vi "AbelFcsMain.vi"() -> ()   [LabVIEW 2009]
uses:
  Camera/vi/ccdChipPixels.vi
  Camera/vi/GlobalSetGetConfigureCamera.vi
  Camera/lib/System Files/user.lib/atmcd32d.llb/Shutter_mode typedef.ctl
  Camera/lib/System Files/user.lib/atmcd32d.llb/Shutter_type typedef.ctl
  Variables/GetPicture.vi
  Camera/vi/StopGetPic.vi
  Camera/vi/CamDef.vi
  Variables/GlobalLaserInterface.vi
  Variables/patternImg.vi
  <vilib>/vision/Image Controls.llb/IMAQ Rounding Mode.ctl
  Variables/GlobalConAxisPI.vi
  Variables/GlobalCameraHandle.vi
  <vilib>/vision/Pattern Matching.llb/IMAQ Match Range Setting.ctl
  <vilib>/vision/Pattern Matching.llb/IMAQ Curve Parameters.ctl
panel:
  out "subarray":dbl[](array[numeric])
  in  "Settings (GeometricMatching)":T3 {"Curve Parameters"."Extraction Mode" items=["Normal", "Uniform Regions"]; "Curve Parameters"."Edge Filter Size" items=["Fine", "Normal", "Contour Tracing"]; "Curve Parameters"."Max Endpoint Gap" min=0; "Curve Parameters"."Col Search Step Size" min=1 max=255 step=1; "Curve Parameters"."Row Search Step Size" min=1 max=255 step=1; "Curve Parameters"."Min Length" min=0; "Curve Parameters"."Edge Threshold" min=1 max=350 step=1; "Range Settings"."Max" format="%.2f"; "Range Settings"."Min" format="%.2f"; "Range Settings"."Match Constraints" items=["Rotation Angle (degrees)", "Scale Factor (%)", "Occlusion (%)"]; "Adv. Geometric Match Options 2"."Setup Data Item" items=["Curve Extraction Mode", "Curve Edge Threshold", "Curve Edge Filter Size", "Min Curve Length", "Curve Row Search Step Size", "Curve Col Search Step Size", "Curve Max Endpoint Gap", "Extract Closed Curves", "Enable Subpixel Curve Extraction", "Enable Correlation Score", "Enable Subpixel Accuracy", "Subpixel Iterations", "Subpixel Tolerance", "Initial Match List Length", "Enable Target Template Curve Score", "Min Match Separation Distance", "Min Match Separation Angle", "Min Match Separation Scale", "Max Match Overlap", "Enable Coarse Result", "Enable Calibration Support", "Enable Contrast Reversal", "Search Strategy", "Refinement Match Factor", "Subpixel Match Factor"]}
  in  "Tab Control":T4(tab)
  out "Histogram":i32[][](graph)
  out "Trace":i32[][](graph)
  out "Point":dbl[][](graph)
  out "Image Out":T5(plugin-control)
  out "Image Number":u32
  out "acquired FPS":dbl
  out "Image":i32[][](graph)
  out "AM image":T5(plugin-control)
  out "Number of Particles":i32
  out "Image 2":dbl[][](graph)
  out "Auto Measure Points":i32
  out "NxtAutMesPoint":i32
  out "Pattern":dbl[][](array[numeric])
  out "X Steps":dbl
  out "3dAbelFcs":bool
  out "Y Steps":dbl
  out "Z Steps":dbl
  out "concatenated string":string
  out "Global Stop":bool
  out "Stop Measurement":bool
  in  "DeviceTabs":T6(tab)
  in  "WS File Tree":string(tree)
  out "Workspace":path
  in  "New MSW":bool
  in  "Open MSW":bool
  in  "Sample description":string
  in  "Save Files":bool
  out "Last Image File No":i32
  in  "Get Position":bool
  in  "Move Stage":bool
  in  "X-Position":dbl caption="X" min=0.0 max=200.0 step=0.1 format="%1.3f um"
  in  "Y-Position":dbl caption="Y" min=0.0 max=200.0 step=0.1 format="%1.3f um"
  in  "Z-Position":dbl caption="Z" min=0.0 max=200.0 step=0.1 format="%1.3f um"
  out "x-position":dbl format="%.3f"
  out "y-position":dbl format="%.3f"
  out "z-position":dbl format="%.3f"
  in  "CFD Settings":T7
  in  "Laser  Profile":string
  in  "Auto Exposure::Mode":u32(ring) items=["Relative", "Ignored"]
  in  "Brightness::Mode":u32(ring) items=["Relative", "Ignored"]
  in  "Gain::Mode":u32(ring) items=["Absolute", "Auto", "Relative", "Ignored"]
  in  "Gamma::Mode":u32(ring) items=["Relative", "Off", "Ignored"]
  in  "Shutter::Mode":u32(ring) items=["Auto", "Relative", "Ignored"]
  in  "Trigger::Trigger Activation":u32(ring) items=["Level Low", "Level High"]
  in  "Trigger::Trigger Mode":u32(ring) items=["Mode 0", "Mode 1", "Mode 15", "Off"]
  in  "Trigger Delay::Mode":u32(ring) items=["Absolute", "Relative", "Off", "Ignored"]
  in  "Brightness::Value":dbl min=0.0 max=1023.0 step=1.0
  in  "Shutter::Value":dbl min=1.0 max=4095.0 step=1.0
  in  "Auto Exposure::Value":dbl min=50.0 max=205.0 step=1.0
  in  "Gain::Value":dbl min=0.0 max=680.0 step=1.0
  in  "Trigger::Trigger Parameter":u32 max=0
  in  "Get Temperature":bool
  in  "SET CCD":bool
  in  "OPEN SHUTER":bool
  in  "Close":bool
  in  "Gain":bool
  in  "Start":bool
  in  "Stop":bool
  in  "Exposure":bool
  in  "Set Temperature":bool
  in  "duty cycle":dbl format="%.6f"
  in  "frequency":dbl format="%.6f"
  in  "PI SystemNumber":i32
  in  "Image Measurent Parameters":T8
  in  "Measurement Tab Control":T9(tab)
  in  "SCANNER EMERGENCY":bool
  in  "Stop Program":bool
  out "Task":T10(ring)
  in  "Point Defocussed Cam":bool
  in  "Adjustment":bool
  in  "Laser pulse duration":i32[](array[numeric]) min=2 max=100000 step=1 format="%d µs"
  in  "Measurement Time":i32 min=10 format="%.0d s"
  in  "Point Measurement":bool
  out "Counts":u32[](array[numeric])
  in  "Axis":enum32{"x-y", "x-z", "y-x", "y-z", "z-x", "z-y"}(ring)
  in  "Picture size 2":dbl min=0.1 max=200.0 format="%1.1f um"
  in  "Picture size":dbl min=0.1 max=200.0 format="%1.1f um"
  in  "Pixel time":dbl min=0.1 max=100.0 step=0.1 format="%.1f ms"
  in  "Resolution":dbl min=0.01 max=10.0 step=0.01 format="%.2f µm"
  out "Measure. time":dbl format="%7.1f s"
  in  "Aquire Image":bool
  out "y":i16
  out "x":i16
  in  "Save Color Image":bool
  in  "Cam (Defocused)":bool
  in  "How long?":bool
  out "Estimated Time (h)":dbl
  in  "Mesaurement Time (Sec) / Step":dbl
  in  "Start 3D FCS Abel Scan":bool
  in  "FCS Point Measurement":bool
  in  "Z Stepsize":dbl
  in  "Y Stepsize":dbl
  in  "X Stepsize":dbl
  in  "Z End":dbl
  in  "Y End":dbl
  in  "X End":dbl
  in  "Z Start":dbl
  in  "Y Start":dbl
  in  "X Start":dbl
  in  "Find Mols":bool
  in  "Filter":bool
  in  "Remove Outliers":i32
  in  "Exclude / Include X":bool
  in  "X Start 2":dbl
  in  "X End 2":dbl
  in  "Exclude / Include Y":bool
  in  "Y Start 2":dbl
  in  "Y End 2":dbl
  in  "Measurement Parameter 1":T11 items=["Center of Mass X", "Center of Mass Y", "First Pixel X", "First Pixel Y", "Bounding Rect Left", "Bounding Rect Top", "Bounding Rect Right", "Bounding Rect Bottom", "Max Feret Diameter Start X", "Max Feret Diameter Start Y", "Max Feret Diameter End X", "Max Feret Diameter End Y", "Max Horiz. Segment Length Left", "Max Horiz. Segment Length Right", "Max Horiz. Segment Length Row", "-", "Bounding Rect Width", "Bounding Rect Height", "Bounding Rect Diagonal", "Perimeter", "Convex Hull Perimeter", "Holes' Perimeter", "Max Feret Diameter", "Equivalent Ellipse Major Axis", "Equivalent Ellipse Minor Axis", "Equivalent Ellipse Minor Axis (Feret)", "Equivalent Rect Long Side", "Equivalent Rect Short Side", "Equivalent Rect Diagonal", "Equivalent Rect Short Side (Feret)", "Average Horiz. Segment Length", "Average Vert. Segment Length", "Hydraulic Radius", "Waddel Disk Diameter", "-", "Area", "Holes' Area", "Particle & Holes' Area", "Convex Hull Area", "Image Area", "-", "Number of Holes", "Number of Horiz. Segments", "Number of Vert. Segments", "-", "Orientation", "Max Feret Diameter Orientation", "-", "% Area/Image Area", "% Area/(Particle & Holes' Area)", "Ratio of Equivalent Ellipse Axes", "Ratio of Equivalent Rect Sides", "-", "Elongation Factor", "Compactness Factor", "Heywood Circularity Factor", "Type Factor", "-", "Sum X", "Sum Y", "Sum XX", "Sum XY", "Sum YY", "Sum XXX", "Sum XXY", "Sum XYY", "Sum YYY", "-", "Moment of Inertia XX", "Moment of Inertia XY", "Moment of Inertia YY", "Moment of Inertia XXX", "Moment of Inertia XXY", "Moment of Inertia XYY", "Moment of Inertia YYY", "Norm. Moment of Inertia XX", "Norm. Moment of Inertia XY", "Norm. Moment of Inertia YY", "Norm. Moment of Inertia XXX", "Norm. Moment of Inertia XXY", "Norm. Moment of Inertia XYY", "Norm. Moment of Inertia YYY", "Hu Moment 1", "Hu Moment 2", "Hu Moment 3", "Hu Moment 4", "Hu Moment 5", "Hu Moment 6", "Hu Moment 7"]
  in  "Range Lower Value Par 1":dbl
  in  "Range Upper Value  Par 1":dbl
  in  "Ex/In Par 1":bool
  in  "Measurement Parameter 2":T11 items=["Center of Mass X", "Center of Mass Y", "First Pixel X", "First Pixel Y", "Bounding Rect Left", "Bounding Rect Top", "Bounding Rect Right", "Bounding Rect Bottom", "Max Feret Diameter Start X", "Max Feret Diameter Start Y", "Max Feret Diameter End X", "Max Feret Diameter End Y", "Max Horiz. Segment Length Left", "Max Horiz. Segment Length Right", "Max Horiz. Segment Length Row", "-", "Bounding Rect Width", "Bounding Rect Height", "Bounding Rect Diagonal", "Perimeter", "Convex Hull Perimeter", "Holes' Perimeter", "Max Feret Diameter", "Equivalent Ellipse Major Axis", "Equivalent Ellipse Minor Axis", "Equivalent Ellipse Minor Axis (Feret)", "Equivalent Rect Long Side", "Equivalent Rect Short Side", "Equivalent Rect Diagonal", "Equivalent Rect Short Side (Feret)", "Average Horiz. Segment Length", "Average Vert. Segment Length", "Hydraulic Radius", "Waddel Disk Diameter", "-", "Area", "Holes' Area", "Particle & Holes' Area", "Convex Hull Area", "Image Area", "-", "Number of Holes", "Number of Horiz. Segments", "Number of Vert. Segments", "-", "Orientation", "Max Feret Diameter Orientation", "-", "% Area/Image Area", "% Area/(Particle & Holes' Area)", "Ratio of Equivalent Ellipse Axes", "Ratio of Equivalent Rect Sides", "-", "Elongation Factor", "Compactness Factor", "Heywood Circularity Factor", "Type Factor", "-", "Sum X", "Sum Y", "Sum XX", "Sum XY", "Sum YY", "Sum XXX", "Sum XXY", "Sum XYY", "Sum YYY", "-", "Moment of Inertia XX", "Moment of Inertia XY", "Moment of Inertia YY", "Moment of Inertia XXX", "Moment of Inertia XXY", "Moment of Inertia XYY", "Moment of Inertia YYY", "Norm. Moment of Inertia XX", "Norm. Moment of Inertia XY", "Norm. Moment of Inertia YY", "Norm. Moment of Inertia XXX", "Norm. Moment of Inertia XXY", "Norm. Moment of Inertia XYY", "Norm. Moment of Inertia YYY", "Hu Moment 1", "Hu Moment 2", "Hu Moment 3", "Hu Moment 4", "Hu Moment 5", "Hu Moment 6", "Hu Moment 7"]
  in  "Range Lower Value Par 2":dbl
  in  "Range Upper Value Par 2":dbl
  in  "Ex/In Par 2":bool
  in  "Square/Hexa":bool
  in  "Connectivity 4/8":bool
  in  "Manual":bool
  in  "Focuswidth":dbl
  in  "Mode":enum16{"Gauss", "Radial", "Azimuthal"}(ring)
  in  "Detection Modus":u16(ring) items=["Pattern", "Heuristic"]
  in  "NA":dbl
  in  "TSH":dbl min=0.0 max=1.0 step=0.01
  in  "Auto Defocussed Cam":bool
  in  "Autopoint-Autofocus Z":bool
  in  "Auto Measurement Time (ms)":i32 caption="Measurement Time (s)" min=10
  out "Auto Meas Progress":i32(slide) caption="Point 34 / 34"
  in  "Auto Meas":bool
  out "Active pt3":path
  out "Buffer Overrun":bool
  out "Running":bool
  # "Range"
  # "Scanner Position"
  # "Point Measurement Settings"
  # "Start Experiment"
  # "Estimated Mesaurement Time"
  # "Image Scan Settings"
  # "Save as png"
  # "Pixel"
  # "Define the 3D Space and Stepwith of your Experiment"
  # "Time of the Experiment"
  # "Check What to Mesaure"
  # "Start Your Experiment here"
  # "Lifetime Mesaurement Time on each Position"
  # "Define Search Area"
  # "Define Detection Parameters"
  # "Exact Matching"
  # "Operation"
  # "Show Progress"
  # "Automated Mesaurement on Single Molecule Coordinates on the  2D Frame"
  # "Start Your Experiment here"
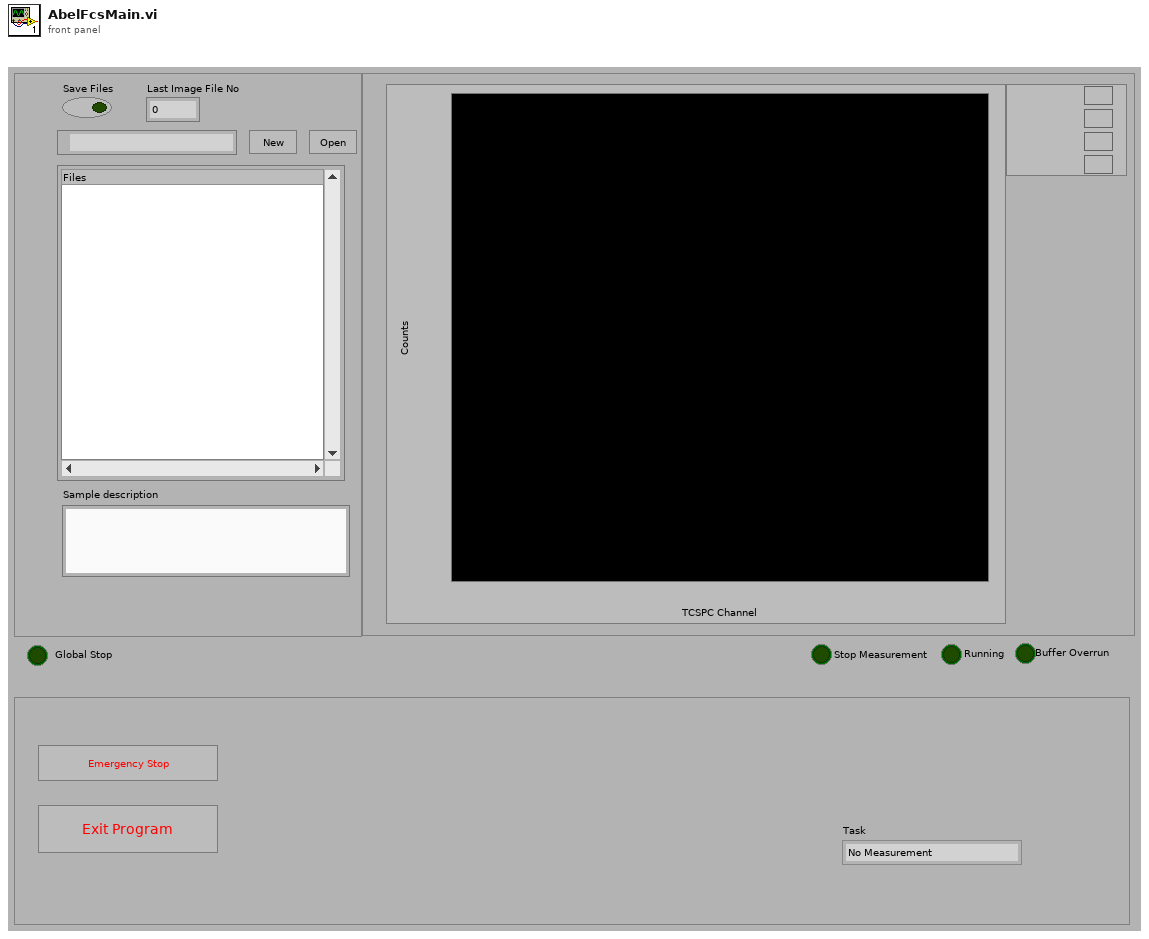
[diagram p1: front panel]
types:
  T1 = typedef "IMAQ Curve Parameters.ctl" = cluster{"Extraction Mode":u32, "Edge Threshold":i32, "Edge Filter Size":u32, "Min Length":i32, "Row Search Step Size":i32, "Col Search Step Size":i32, "Max Endpoint Gap":i32, "Closed":bool, "Subpixel":bool}
  T2 = typedef "IMAQ Match Range Setting.ctl" = cluster{"Match Constraints":u32, "Min":dbl, "Max":dbl}
  T3 = cluster{"Curve Parameters":T1, "Match Mode":cluster{"Rotation":bool, "Scale":bool, "Occlusion":bool, "Reserved":bool, "Reserved":bool, "Reserved":bool}, "Range Settings":T2[], "Number of Matches":i32, "Minimum Match Score":sgl, "SubPixel Accuracy":bool, "Adv. Geometric Match Options 2":cluster{"Setup Data Item":u16, "Item Value":dbl}[]}
  T4 = enum32{"TCSPC Histogram", "Trace", "CCD", "Backreflection", "Image", "AutoMesaurement"}
  T5 = typedef "IMAQ Image.ctl" = refnum<image>
  T6 = enum32{"Workspace", "Scanner", "HHL", "Video", "CCD", "Laser2"}
  T7 = cluster{"Sync Level":i32, "Sync ZeroX":i32, "Sync Offset":i32, "Chan Settings":cluster{"CHx Level":i32, "CHx ZeroX":i32, "CHx Offset":i32}[]}
  T8 = cluster{"Position":cluster{"X-Position":dbl, "Y-Position":dbl, "Z-Position":dbl}, "Axis 1 Pixels":dbl, "Axis 2 Pixels":dbl, "Axis":i32, "Resolution":dbl, "PixelTime":dbl, "Laser pulses":i32}
  T9 = enum32{"Main ", "Point Measurement", "Aquire Image (Area Scan)", "3D Grid FCS CCD", "Search Molecules", "AutoMode"}
  T10 = enum16{"No Measurement", "Aquire Image", "Point Measurement", "Multi Measurement", "Save Color Image", "Find Single Mol.", "Auto Measurement Control", "Auto Point", "Aquire Line Scan", "Grid Measurement", "Trapping", "Move Scanner"}
  T11 = typedef "Particle Parameters" = i32
  T12 = cluster{"Dev":i32, "SerNo":string, "HW_Model":string, "HW_Partno":string}[]
  T13 = enum16{"No Measurement", "Aquire Image", "Point Measurement", "Multi Measurement", "Save Color Image"}
  T14 = enum16{"No Measurement", "Aquire Image", "Point Measurement", "Multi Measurement", "Save Color Image", "Find Single Mol.", "Auto Measurement Control", "Auto Point"}
  T15 = enum16{"No Measurement", "Aquire Image", "Point Measurement", "Multi Measurement", "Save Color Image", "Find Single Mol."}
  T16 = enum16{"Get (Default)", "Set Workspace", "Append File", "Change Comment"}
  T17 = typedef "Shutter_type typedef.ctl" = enum16{"TTL Low", "TTL High"}
  T18 = typedef "Shutter_mode typedef.ctl" = enum16{"Auto", "Open", "Close"}
  T19 = cluster{"File No":i32, "File Path":path, "Parent File":i32, "File Type":enum16{"unknown", "pt3 File", "png Image", "bmp Image"}, "Measurement Type":enum16{"not a pt3 File", "Image File", "Point Measurement", "Auto Point", "Line Scan", "Grid Scan"}, "Upper Left":cluster{"x-Position":dbl, "y-Position":dbl, "z-Position":dbl}, "Pixels":dbl[], "Resolution":dbl, "Scan Axis":enum32{"x-y", "x-z", "y-x", "y-z", "z-x", "z-y"}, "PixelTime":dbl}[]
  T20 = cluster{"File No":i32, "File Path":path, "Parent File":i32, "File Type":enum16{"unknown", "pt3 File", "png Image", "bmp Image"}, "Measurement Type":enum16{"not a pt3 File", "Image File", "Point Measurement", "Auto Point", "Line Scan", "Grid Scan"}, "Upper Left":cluster{"x-Position":dbl, "y-Position":dbl, "z-Position":dbl}, "Pixels":i32[], "Scan Axis":enum32{"x-y", "x-z", "y-x", "y-z", "z-x", "z-y"}, "Resolution":dbl, "PixelTime":dbl}[]
  T21 = cluster{"File No":i32, "File Path":path, "Parent File":i32, "File Type":enum16{"unknown", "pt3 File", "png Image", "bmp Image"}, "Measurement Type":enum16{"not a pt3 File", "Image File", "Point Measurement", "Auto Point", "Line Scan", "Grid Scan"}, "Upper Left":cluster{"x-Position":dbl, "y-Position":dbl, "z-Position":dbl}, "Pixels":i32[], "Resolution":dbl, "Scan Axis":enum32{"x-y", "x-z", "y-z"}, "PixelTime":dbl}[]
  T22 = cluster{"Files in Workspace[0]":cluster{"File No":i32, "File Path":path, "Parent File":i32, "File Type":enum16{"unknown", "pt3 File", "png Image", "bmp Image"}, "Measurement Type":enum16{"not a pt3 File", "Image File", "Point Measurement", "Auto Point", "Line Scan", "Grid Scan"}, "Upper Left":cluster{"x-Position":dbl, "y-Position":dbl, "z-Position":dbl}, "Pixels":i32[], "Scan Axis":enum32{"x-y", "x-z", "y-x", "y-z", "z-x", "z-y"}, "Resolution":dbl, "PixelTime":dbl}, "Files in Workspace[1]":cluster{"File No":i32, "File Path":path, "Parent File":i32, "File Type":enum16{"unknown", "pt3 File", "png Image", "bmp Image"}, "Measurement Type":enum16{"not a pt3 File", "Image File", "Point Measurement", "Auto Point", "Line Scan", "Grid Scan"}, "Upper Left":cluster{"x-Position":dbl, "y-Position":dbl, "z-Position":dbl}, "Pixels":i32[], "Scan Axis":enum32{"x-y", "x-z", "y-x", "y-z", "z-x", "z-y"}, "Resolution":dbl, "PixelTime":dbl}, "Files in Workspace[2]":cluster{"File No":i32, "File Path":path, "Parent File":i32, "File Type":enum16{"unknown", "pt3 File", "png Image", "bmp Image"}, "Measurement Type":enum16{"not a pt3 File", "Image File", "Point Measurement", "Auto Point", "Line Scan", "Grid Scan"}, "Upper Left":cluster{"x-Position":dbl, "y-Position":dbl, "z-Position":dbl}, "Pixels":i32[], "Scan Axis":enum32{"x-y", "x-z", "y-x", "y-z", "z-x", "z-y"}, "Resolution":dbl, "PixelTime":dbl}, "Files in Workspace[3]":cluster{"File No":i32, "File Path":path, "Parent File":i32, "File Type":enum16{"unknown", "pt3 File", "png Image", "bmp Image"}, "Measurement Type":enum16{"not a pt3 File", "Image File", "Point Measurement", "Auto Point", "Line Scan", "Grid Scan"}, "Upper Left":cluster{"x-Position":dbl, "y-Position":dbl, "z-Position":dbl}, "Pixels":i32[], "Scan Axis":enum32{"x-y", "x-z", "y-x", "y-z", "z-x", "z-y"}, "Resolution":dbl, "PixelTime":dbl}, "Files in Workspace[4]":cluster{"File No":i32, "File Path":path, "Parent File":i32, "File Type":enum16{"unknown", "pt3 File", "png Image", "bmp Image"}, "Measurement Type":enum16{"not a pt3 File", "Image File", "Point Measurement", "Auto Point", "Line Scan", "Grid Scan"}, "Upper Left":cluster{"x-Position":dbl, "y-Position":dbl, "z-Position":dbl}, "Pixels":i32[], "Scan Axis":enum32{"x-y", "x-z", "y-x", "y-z", "z-x", "z-y"}, "Resolution":dbl, "PixelTime":dbl}, "Files in Workspace[5]":cluster{"File No":i32, "File Path":path, "Parent File":i32, "File Type":enum16{"unknown", "pt3 File", "png Image", "bmp Image"}, "Measurement Type":enum16{"not a pt3 File", "Image File", "Point Measurement", "Auto Point", "Line Scan", "Grid Scan"}, "Upper Left":cluster{"x-Position":dbl, "y-Position":dbl, "z-Position":dbl}, "Pixels":i32[], "Scan Axis":enum32{"x-y", "x-z", "y-x", "y-z", "z-x", "z-y"}, "Resolution":dbl, "PixelTime":dbl}, "Files in Workspace[6]":cluster{"File No":i32, "File Path":path, "Parent File":i32, "File Type":enum16{"unknown", "pt3 File", "png Image", "bmp Image"}, "Measurement Type":enum16{"not a pt3 File", "Image File", "Point Measurement", "Auto Point", "Line Scan", "Grid Scan"}, "Upper Left":cluster{"x-Position":dbl, "y-Position":dbl, "z-Position":dbl}, "Pixels":i32[], "Scan Axis":enum32{"x-y", "x-z", "y-x", "y-z", "z-x", "z-y"}, "Resolution":dbl, "PixelTime":dbl}, "Files in Workspace[7]":cluster{"File No":i32, "File Path":path, "Parent File":i32, "File Type":enum16{"unknown", "pt3 File", "png Image", "bmp Image"}, "Measurement Type":enum16{"not a pt3 File", "Image File", "Point Measurement", "Auto Point", "Line Scan", "Grid Scan"}, "Upper Left":cluster{"x-Position":dbl, "y-Position":dbl, "z-Position":dbl}, "Pixels":i32[], "Scan Axis":enum32{"x-y", "x-z", "y-x", "y-z", "z-x", "z-y"}, "Resolution":dbl, "PixelTime":dbl}, "Files in Workspace[8]":cluster{"File No":i32, "File Path":path, "Parent File":i32, "File Type":enum16{"unknown", "pt3 File", "png Image", "bmp Image"}, "Measurement Type":enum16{"not a pt3 File", "Image File", "Point Measurement", "Auto Point", "Line Scan", "Grid Scan"}, "Upper Left":cluster{"x-Position":dbl, "y-Position":dbl, "z-Position":dbl}, "Pixels":i32[], "Scan Axis":enum32{"x-y", "x-z", "y-x", "y-z", "z-x", "z-y"}, "Resolution":dbl, "PixelTime":dbl}}
  T23 = typedef "LVPoint32TypeDef.ctl" = cluster{"Horizontal":i32, "Vertical":i32}
  T24 = cluster{"Shift":bool, "Ctrl":bool, "Alt":bool, "Cmd":bool, "Opt":bool}
  T25 = enum16{"No Measurement", "Aquire Image", "Point Measurement", "Multi Measurement", "Save Color Image", "Find Single Mol.", "Auto Measurement Control", "Auto Point", "Aquire Line Scan", "Grid Measurement"}
  T26 = enum16{"none", "fast axis", "slow axis", "both axis", ""}
  T27 = enum16{"none", "fast axis", "slow axis", "both", ""}
  T28 = enum16{"target position", "relative position", "actual position", "position error"}
  T29 = enum16{"not a pt3 File", "Image File", "Point Measurement", "Auto Point"}
  T30 = enum16{"unknown", "pt3 File", "png Image", "bmp Image"}
  T31 = typedef "IMAQ Rounding Mode.ctl" = enum16{"Optimize", "Truncate"}
  T32 = cluster{"Measurement Parameter":T11, "Range Lower Value":dbl, "Range Upper Value":dbl, "Range":bool, "Measurement Type":bool}[]
  T33 = enum16{"not a pt3 File", "Image File", "Point Measurement", "Auto Point", "Line Scan"}
  T34 = cluster{"Dev":i32, "SerNo":string, "HW_Model":string, "HW_Partno":string}
  T35 = cluster{"Comment":string, "Binning":i32, "Offset":i32, "AcquisitionTime (ms)":i32, "HardwareSerial":i32, "SyncDivider":i32, "Resolution (ps)":dbl, "CFD Settings":cluster{"Sync Level":i32, "Sync ZeroX":i32, "Sync Offset":i32, "Chan Settings":cluster{"CHx Level":i32, "CHx ZeroX":i32, "CHx Offset":i32}[]}, "ModuleInfo":cluster{"modelcode":i32, "versioncode":i32}[], "BaseResolution (ps)":dbl, "RefClockSource":i32, "ChanInfo":cluster{"CHx Level":i32, "CHx ZeroX":i32, "CHx Offset":i32, "CHx modidx":i32}[], "SyncRate":i32, "InputsEnabled":i64}
  T36 = cluster{"Dimensions":i32, "Time Per Pixel [ms]":dbl, "Acceleration":i32, "Pattern":i32, "X0":sgl, "Y0":sgl, "Z0":dbl, "PixX":i32, "PixY":i32, "PixResol":sgl, "TStartTo":sgl, "TStoptTo":sgl, "TStartFro":sgl, "TStopFro":sgl}
  T37 = cluster{"InpRateFilePos":i64, "StopAfterFilePos":i64}
  T38 = cluster{"X-Position":dbl, "Y-Position":dbl, "Z-Position":dbl}
  T39 = cluster{"File No":i32, "File Path":path, "Parent File":i32, "File Type":enum16{"unknown", "pt3 File", "png Image", "bmp Image"}, "Measurement Type":enum16{"not a pt3 File", "Image File", "Point Measurement", "Auto Point", "Line Scan", "Grid Scan"}, "Upper Left":cluster{"x-Position":dbl, "y-Position":dbl, "z-Position":dbl}, "Pixels":i32[], "Scan Axis":enum32{"x-y", "x-z", "y-z"}, "Resolution":dbl, "PixelTime":dbl}
  T40 = enum16{"not a pt3 File", "Image File", "Point Measurement", "Auto Point", "Line Scan", "Grid Scan"}
  T41 = cluster{"Ident":string, "Format Version":string, "Creator Name":string, "Creator Version":string, "File Time":string, "Comment":string, "Laser":i32, "Binning":i32, "Offset":i32, "AcquisitionTime (ms)":i32, "HardwareSerial":i32, "SyncDivider":i32, "Resolution (ps)":dbl, "Rates":dbl[], "SyncRate":dbl, "CFD Settings":cluster{"Sync Level":i32, "Sync ZeroX":i32, "Sync Offset":i32, "Chan Settings":cluster{"CHx Level":i32, "CHx ZeroX":i32, "CHx Offset":i32}[]}}
  T42 = cluster{"x-Position":dbl, "y-Position":dbl, "z-Position":dbl}
  T43 = typedef "Image Type" = u32
  T44 = cluster{"MesaurementSelection[0]":cluster{"Measurement Parameter":T11, "Range Lower Value":dbl, "Range Upper Value":dbl, "Range":bool, "Measurement Type":bool}, "MesaurementSelection[1]":cluster{"Measurement Parameter":T11, "Range Lower Value":dbl, "Range Upper Value":dbl, "Range":bool, "Measurement Type":bool}, "MesaurementSelection[2]":cluster{"Measurement Parameter":T11, "Range Lower Value":dbl, "Range Upper Value":dbl, "Range":bool, "Measurement Type":bool}, "MesaurementSelection[3]":cluster{"Measurement Parameter":T11, "Range Lower Value":dbl, "Range Upper Value":dbl, "Range":bool, "Measurement Type":bool}, "MesaurementSelection[4]":cluster{"Measurement Parameter":T11, "Range Lower Value":dbl, "Range Upper Value":dbl, "Range":bool, "Measurement Type":bool}, "MesaurementSelection[5]":cluster{"Measurement Parameter":T11, "Range Lower Value":dbl, "Range Upper Value":dbl, "Range":bool, "Measurement Type":bool}, "MesaurementSelection[6]":cluster{"Measurement Parameter":T11, "Range Lower Value":dbl, "Range Upper Value":dbl, "Range":bool, "Measurement Type":bool}, "MesaurementSelection[7]":cluster{"Measurement Parameter":T11, "Range Lower Value":dbl, "Range Upper Value":dbl, "Range":bool, "Measurement Type":bool}, "MesaurementSelection[8]":cluster{"Measurement Parameter":T11, "Range Lower Value":dbl, "Range Upper Value":dbl, "Range":bool, "Measurement Type":bool}}
  T45 = cluster{"Measurement Parameter":T11, "Range Lower Value":dbl, "Range Upper Value":dbl, "Range":bool, "Measurement Type":bool}
  T46 = typedef "IMAQ Point" = cluster{"X":sgl, "Y":sgl}
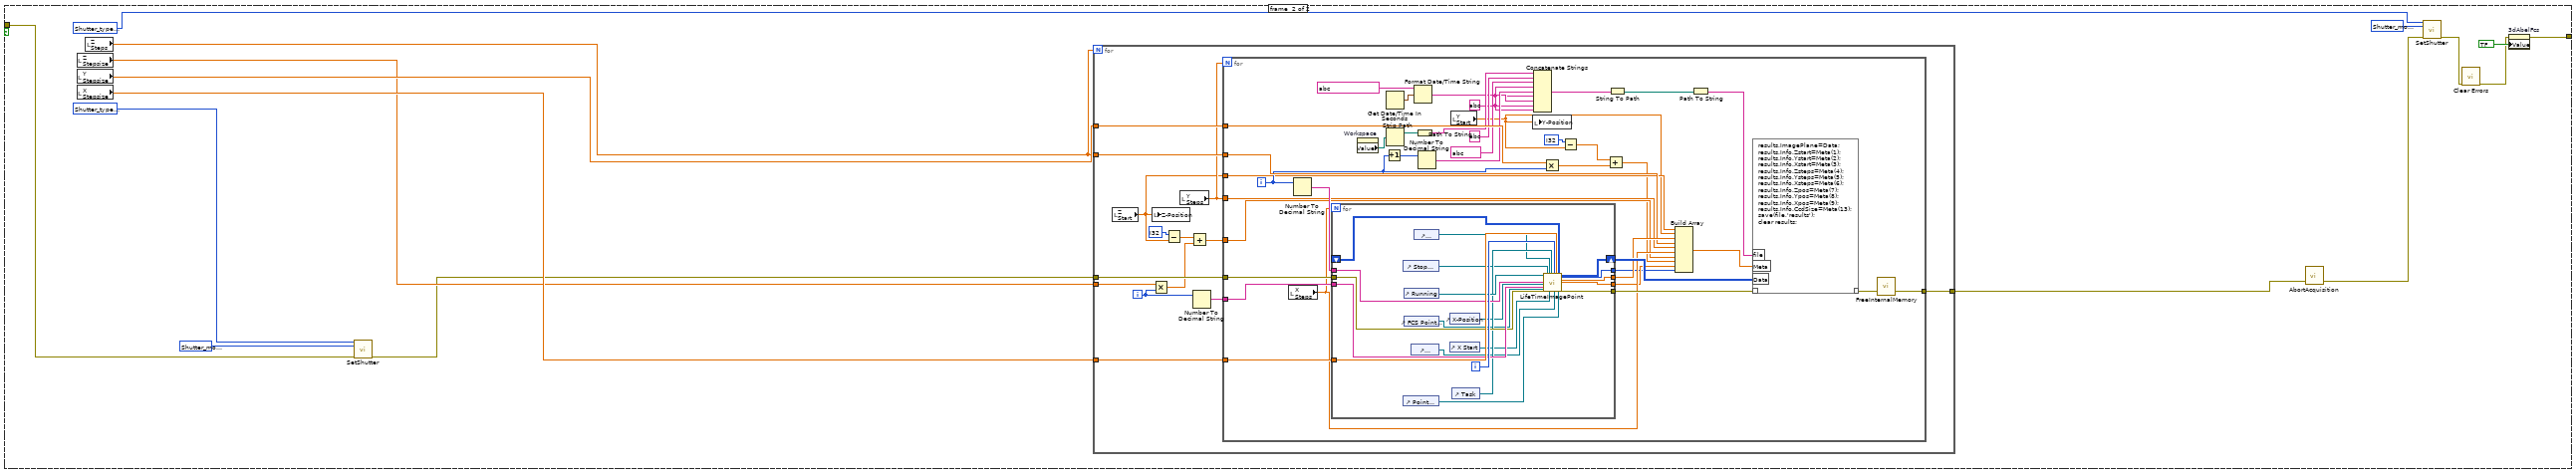
[diagram p2: hidden frame]
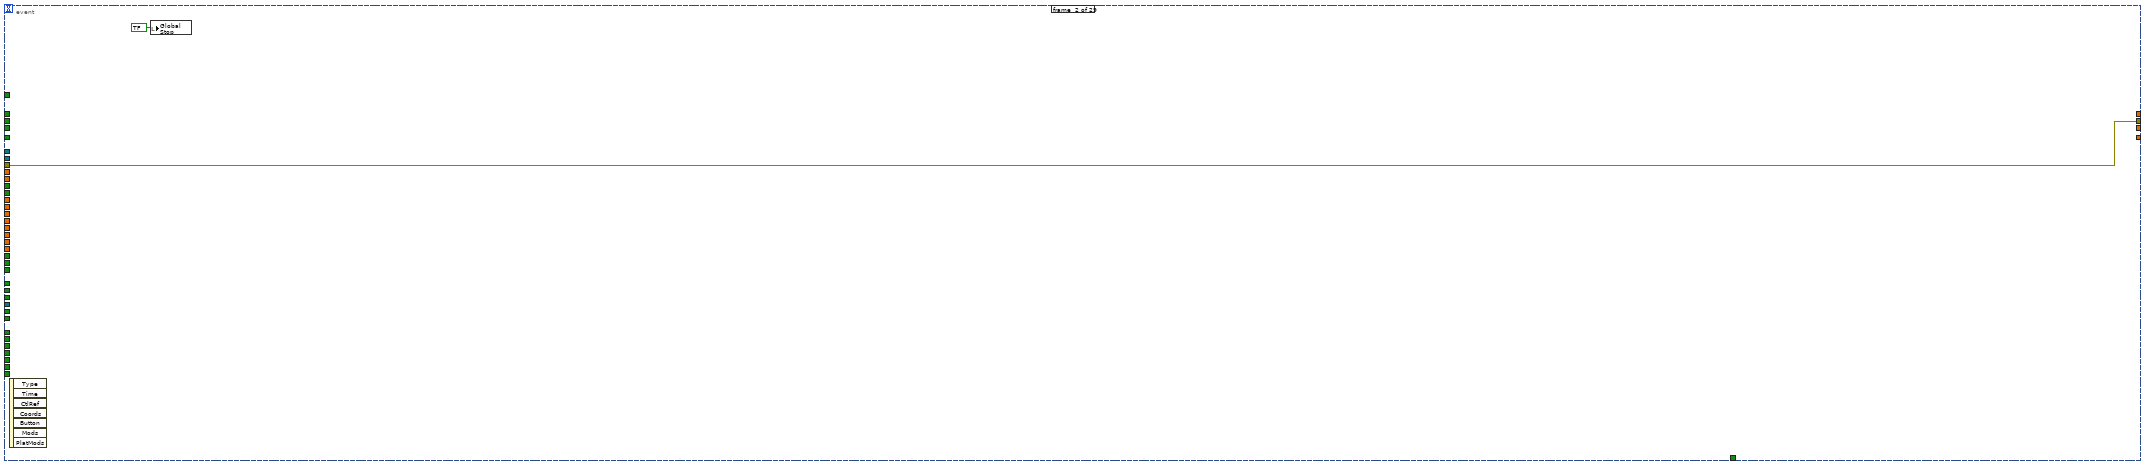
[diagram p3: hidden frame]
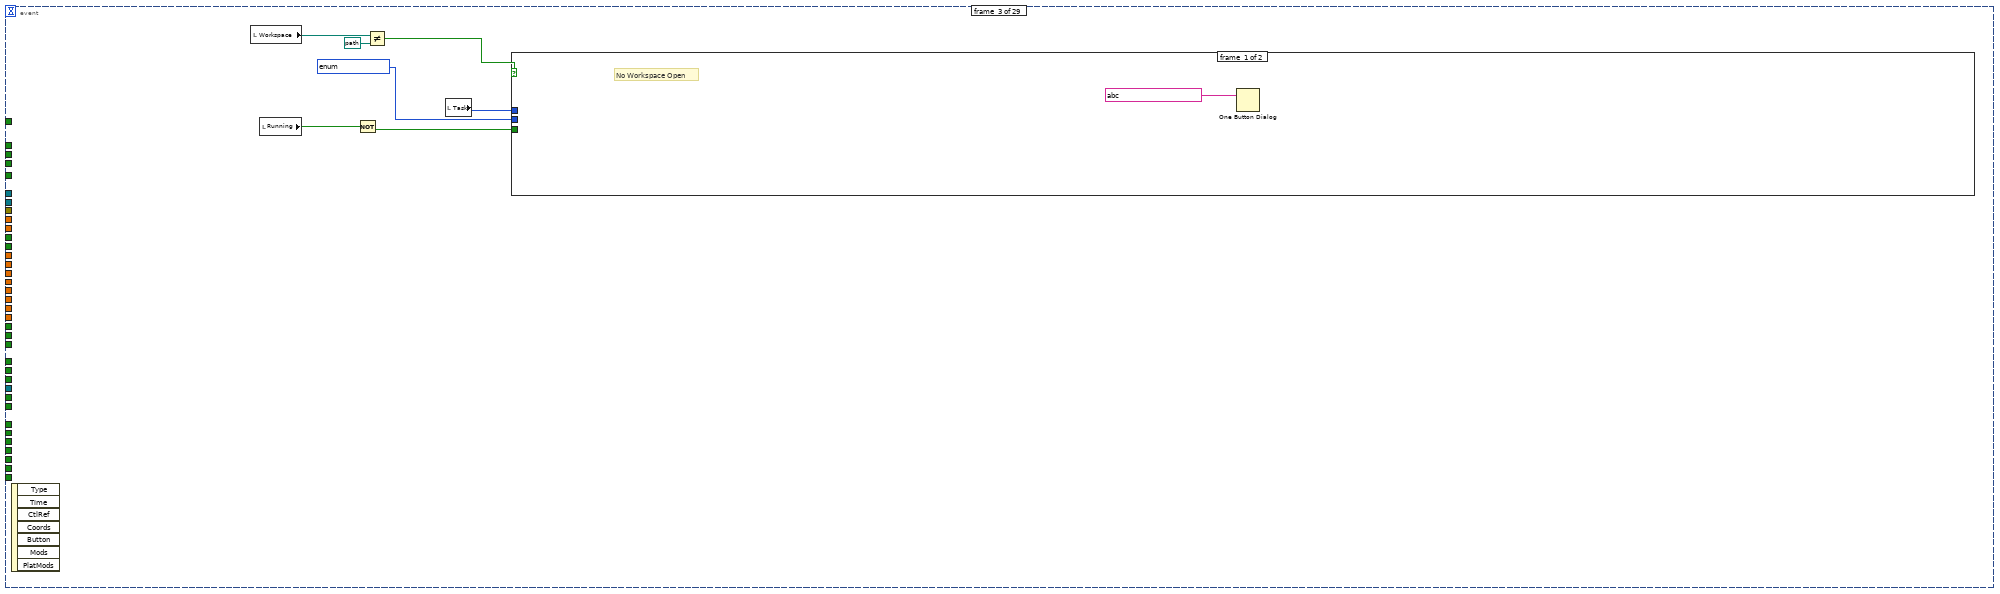
[diagram p4: hidden frame]
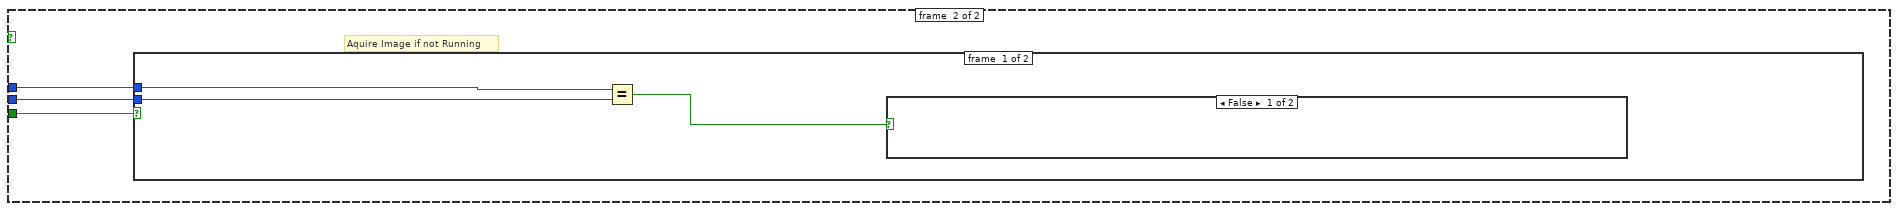
[diagram p5: hidden frame]
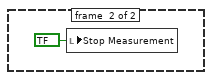
[diagram p6: hidden frame]
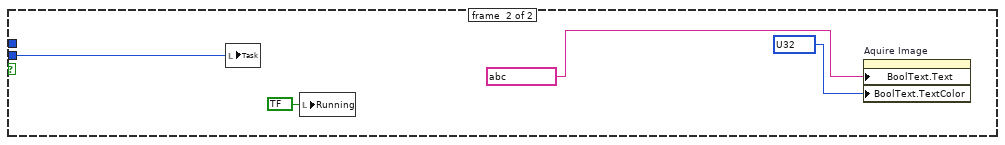
[diagram p7: hidden frame]
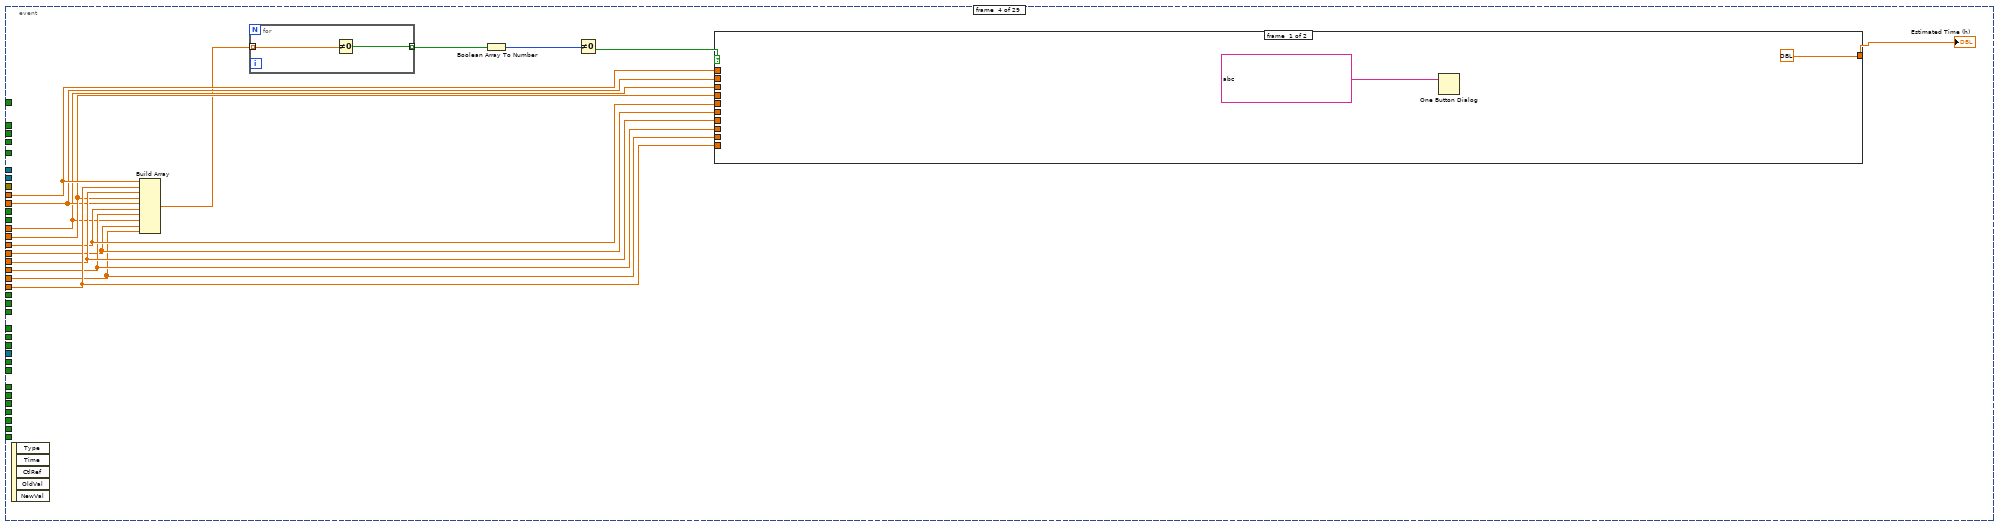
[diagram p8: hidden frame]
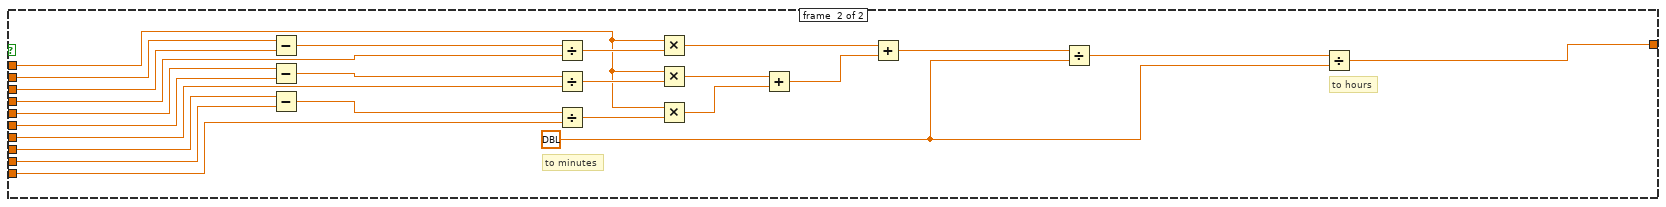
[diagram p9: hidden frame]
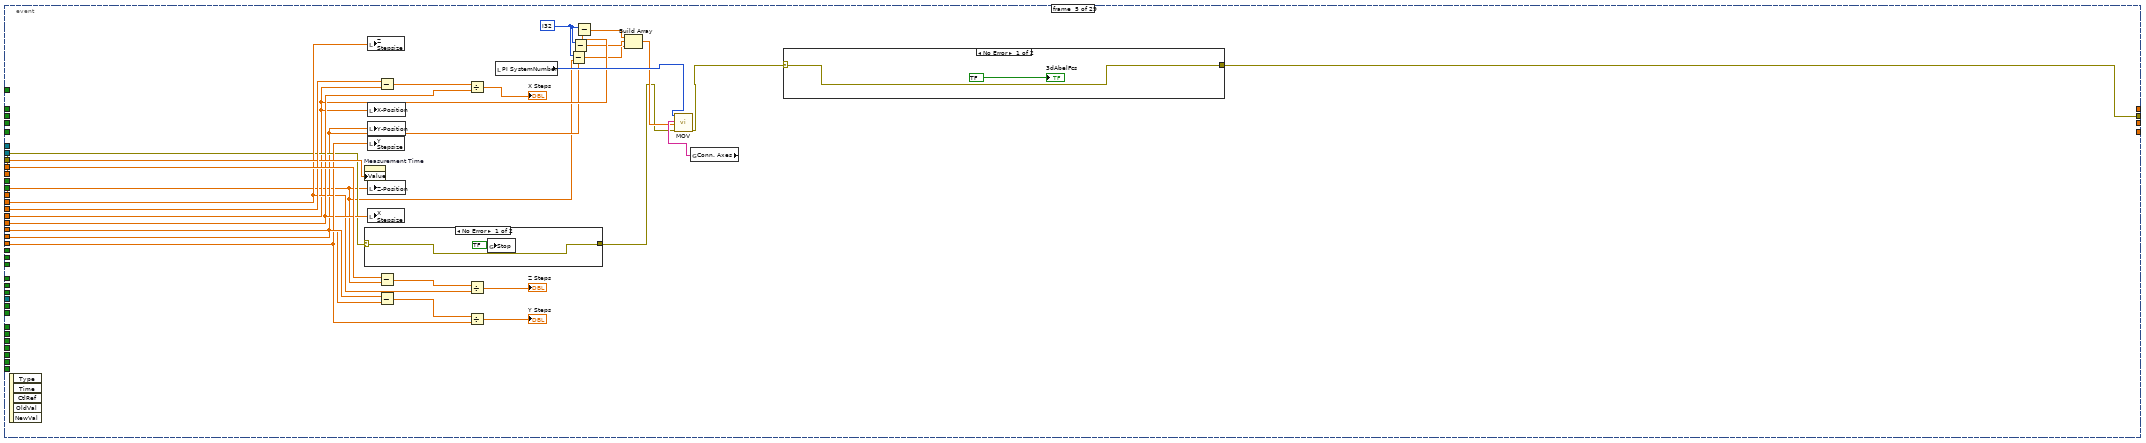
[diagram p10: hidden frame]
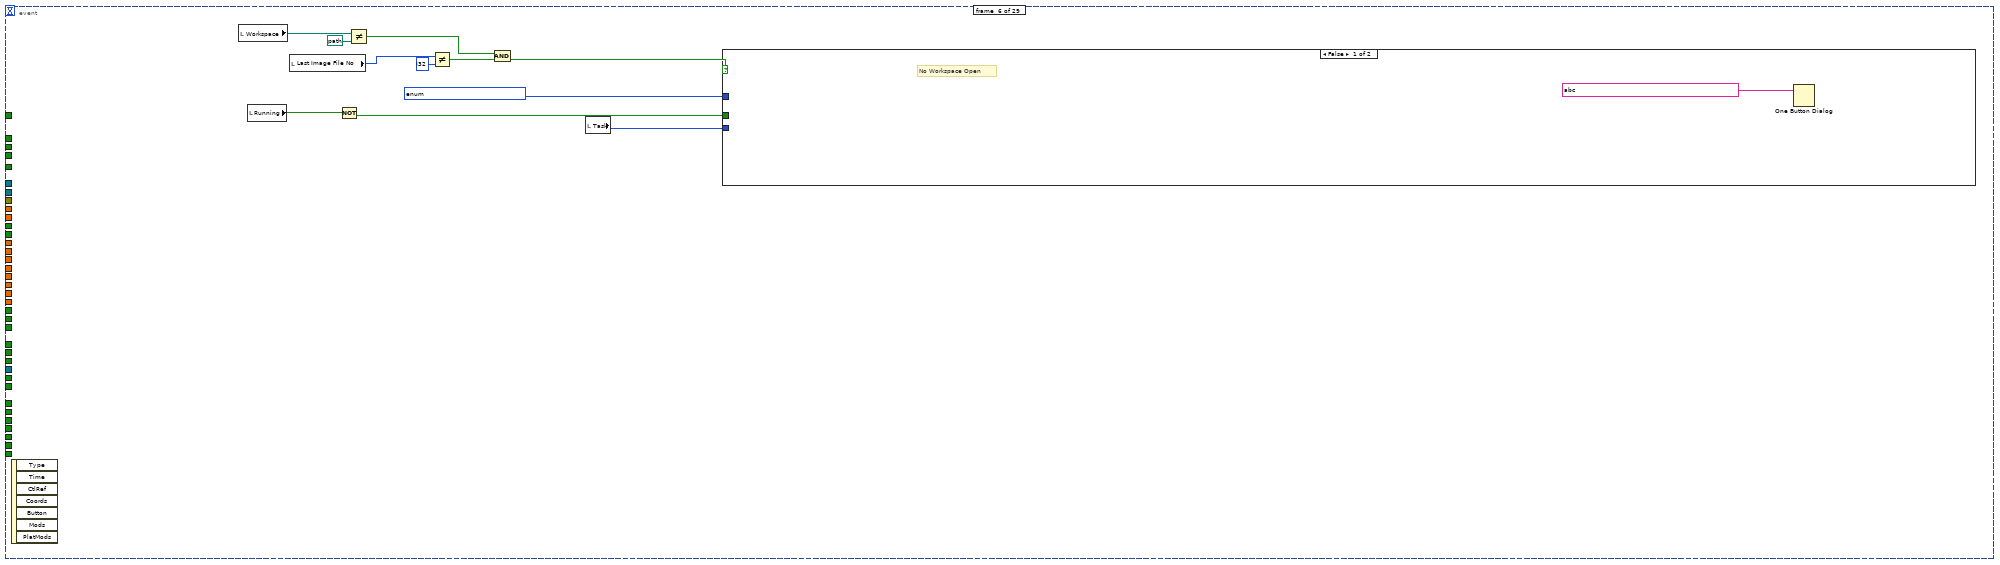
[diagram p13: hidden frame]
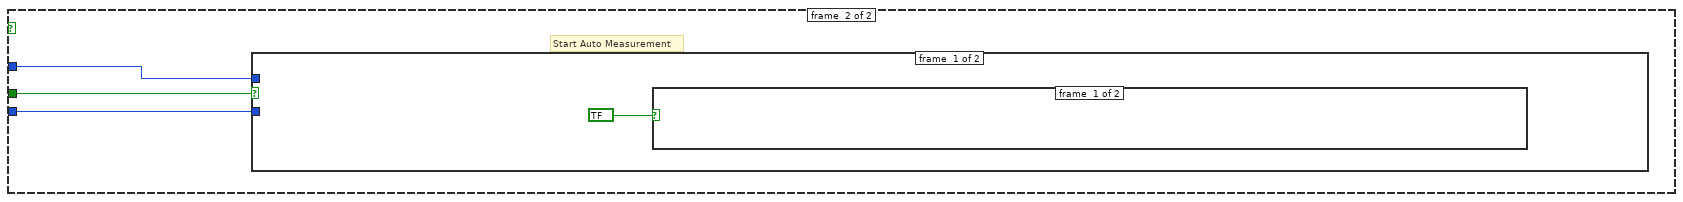
[diagram p14: hidden frame]
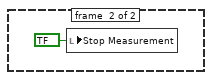
[diagram p15: hidden frame]
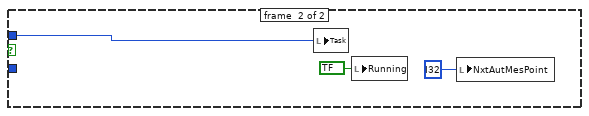
[diagram p16: hidden frame]
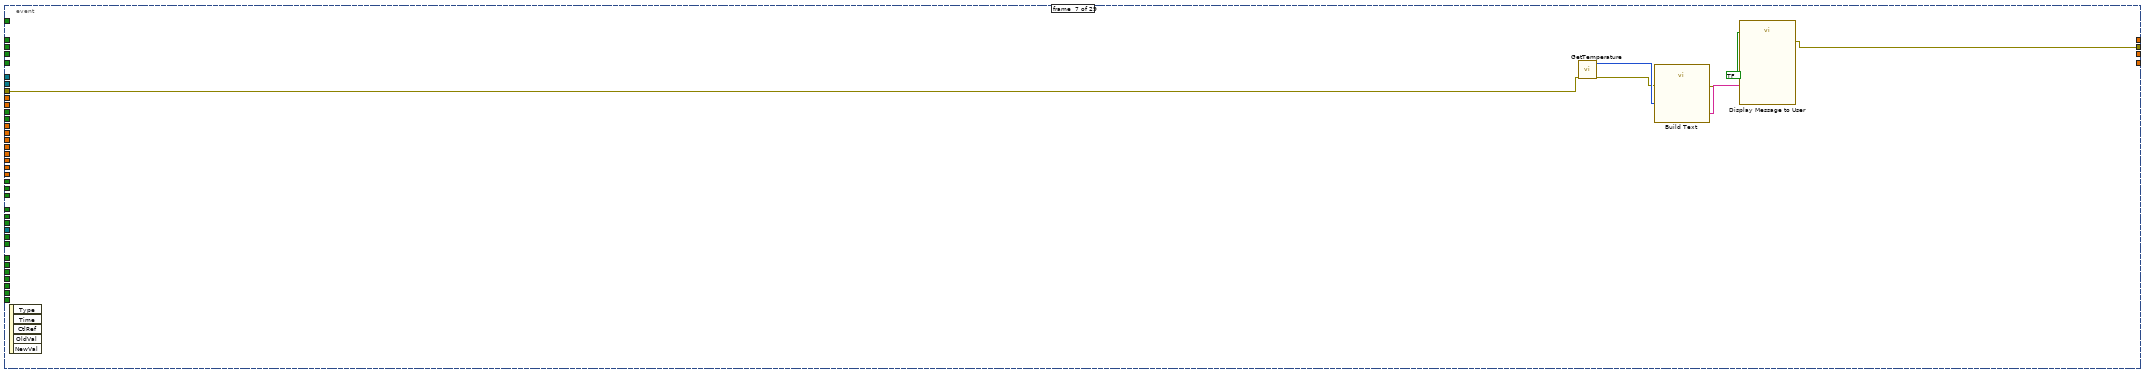
[diagram p17: hidden frame]
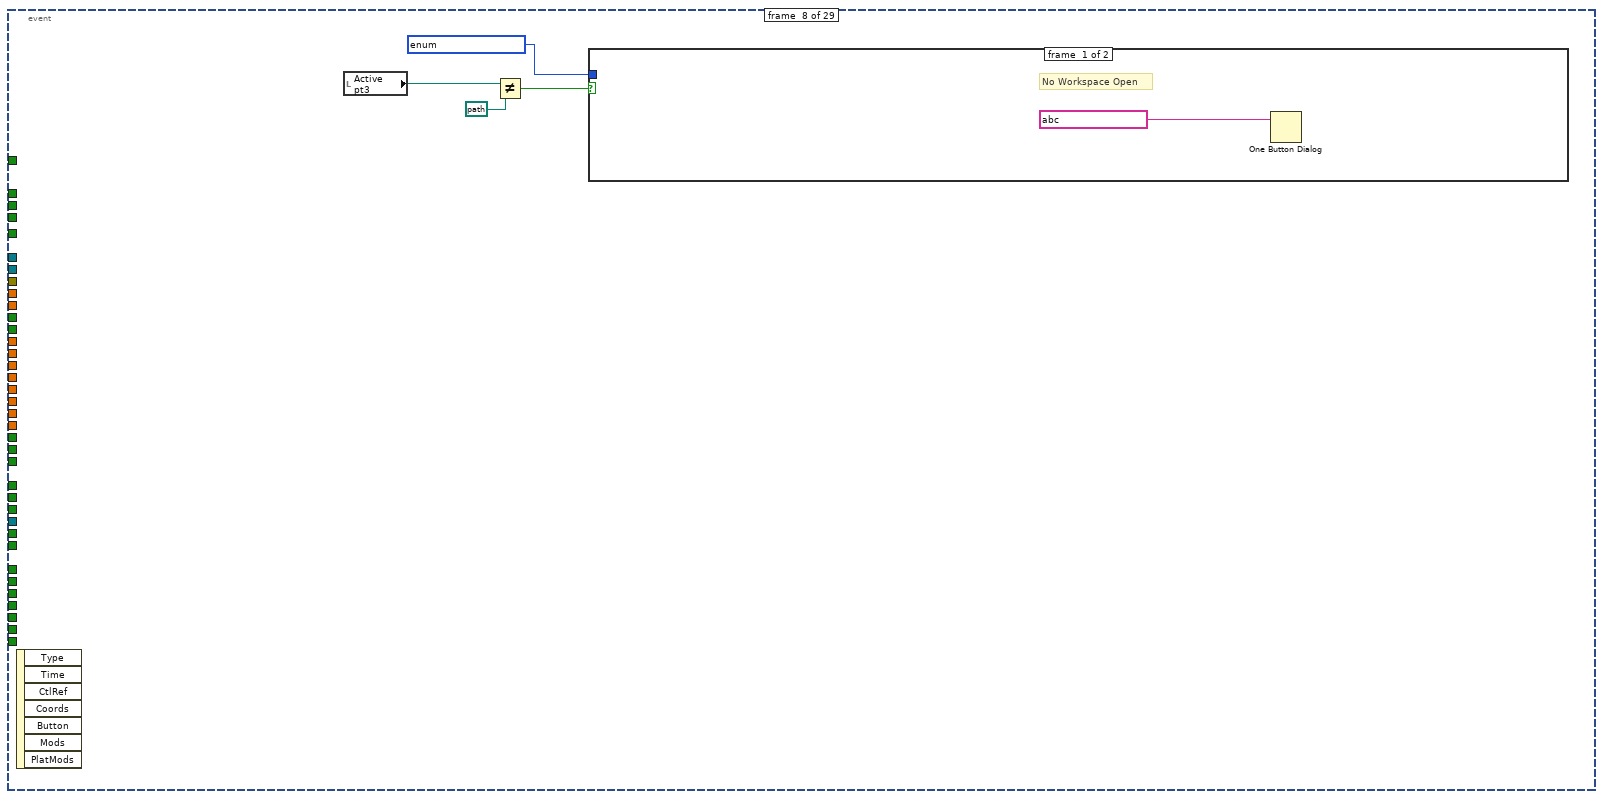
[diagram p18: hidden frame]
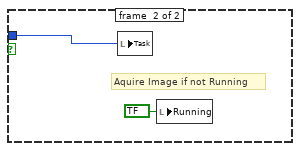
[diagram p19: hidden frame]
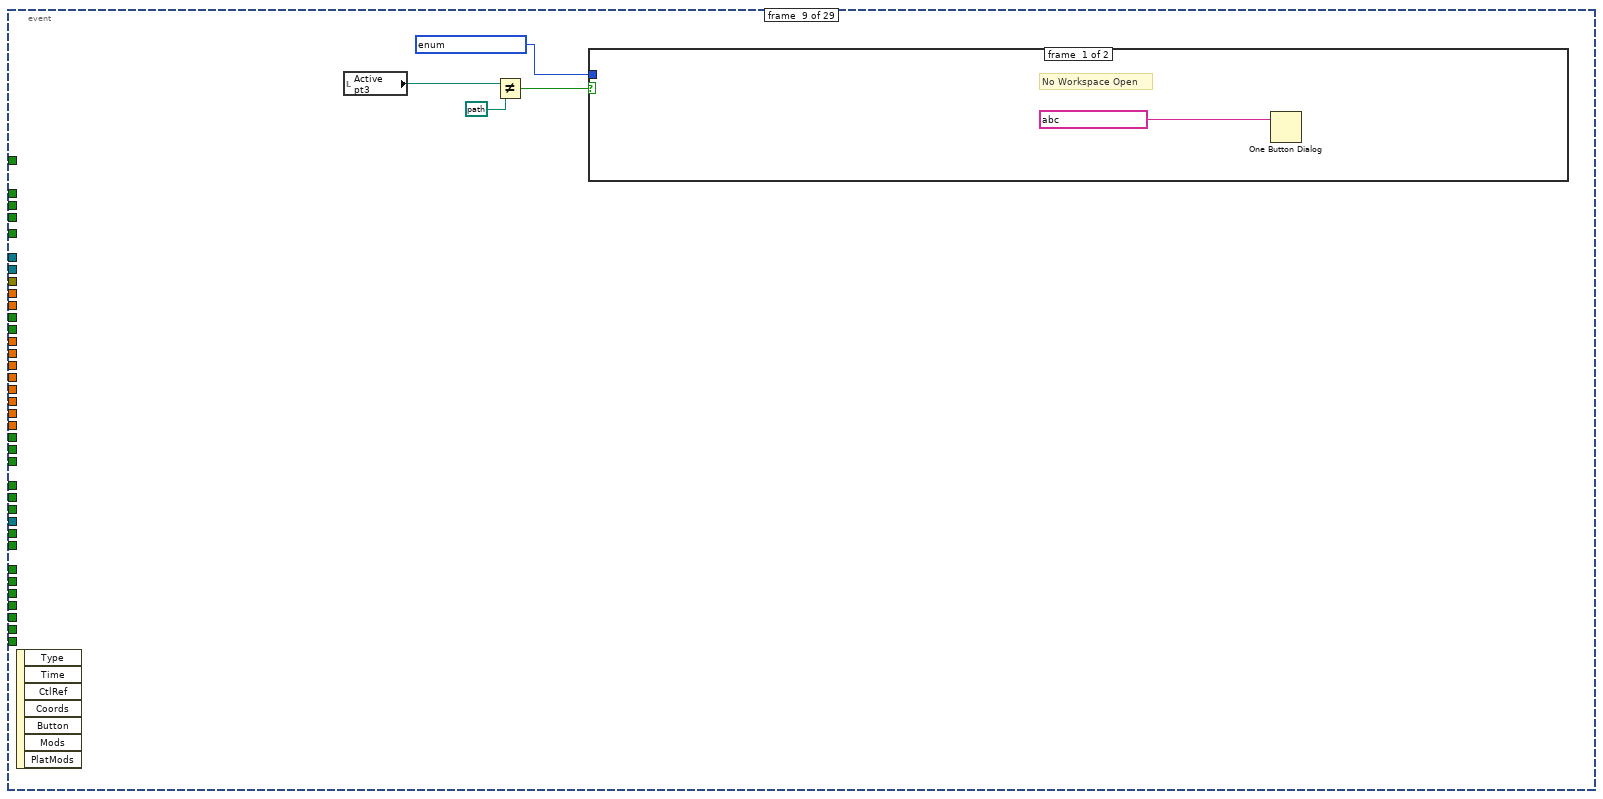
[diagram p20: hidden frame]
diagram:
  n1 = flat-sequence {
    tunnel: [w21] -> w14
    tunnel: errorcluster ? ("error in") -> [w32]
    frame #0 {
      (unwired) dbl ? ("CCD Chip Vertical Start")
      w33 = path ?
      w40 = bool ? ("Global Stop")
      n2 = control-ref of="WS File Tree"() -> (w39:refnum<vi>)
      n3 = global write "GetPicture.vi" "GetPicture"(bool ? ("GetPicture")) -> ()
      n4 = global write "GlobalSetGetConfigureCamera.vi" "gain"(i32 ? ("gain")) -> ()
      n5 = local write "Last Image File No"(i32 ? ("Last Image File No")) -> ()
      n6 = global write "GlobalSetGetConfigureCamera.vi" "Exposure"(sgl ? ("Exposure")) -> ()
      n7 = flat-sequence {
        tunnel: dbl ? ("Vertical Binning") -> [w46]
        tunnel: dbl ? ("CCD Chip Horizontal Start") -> [w45]
        tunnel: dbl ? ("CCD Chip Vertical Start") -> [w41]
        tunnel: dbl ? ("CCD Chip Horizontal End") -> [w44]
        tunnel: dbl ? ("CCD Chip Vertical End") -> [w43]
        tunnel: dbl ? ("Horizontal Binning") -> [w42]
        frame #0 {
          n8 = global write "GlobalSetGetConfigureCamera.vi" "Hbin"(w42) -> ()
          n9 = global write "GlobalSetGetConfigureCamera.vi" "Vbin"(w45) -> ()
          n10 = global write "GlobalSetGetConfigureCamera.vi" "Vbin"(w46) -> ()
          n11 = Subtract(x=w44, y=w45) -> (x-y=w48:dbl)
          n12 = Subtract(x=w43, y=w41) -> (x-y=w47:dbl)
          n13 = global write "ccdChipPixels.vi" "CCD Chip horizontal start"(w41) -> ()
          n14 = global write "ccdChipPixels.vi" "CCD Chip Vertical end"(w43) -> ()
          n15 = global write "ccdChipPixels.vi" "CCD Chip Vertical Start"(w41) -> ()
          n16 = global write "ccdChipPixels.vi" "CCD Chip horizontal end"(w44) -> ()
          n17 = Increment(x=w48) -> (x+1=w50:dbl)
          n18 = Increment(x=w47) -> (x+1=w49:dbl)
          n19 = Multiply(x=w50, y=w49) -> (x*y=w51:dbl)
          n20 = global write "ccdChipPixels.vi" "CCD Chip Size"(w51) -> ()
        }
      }
      n21 = property on="Aquire Image" class="Bool"("BoolText.Text"=string ? ("Caption.Text"), "BoolText.TextColor"=u32 ? ("Boolean Text.Colors:FG Color")) -> ()  [unwired: 2 in, 2 out]
      n22 = property on="Point Measurement" class="Bool"("BoolText.Text"=string ? ("Caption.Text"), "BoolText.TextColor"=u32 ? ("Boolean Text.Colors:FG Color")) -> ()  [unwired: 2 in, 2 out]
      n23 = local write "PI SystemNumber"(i32 ? ("PI SystemNumber")) -> ()
      n24 = global write "GlobalCameraHandle.vi" "CameraHandle"(dbl ? ("CameraHandle")) -> ()
      n25 = call "MTS_ClearWSTree2.vi"("error in"=w32, "Tree Refnum"=w39) -> ("error out"=w21:errorcluster)  [unwired: 8 in, 1 out]
      "Global Stop" <- w40
      "Running" <- w40
      "Buffer Overrun" <- w40
      "Stop Measurement" <- w40
      "Workspace" <- w33
      "Active pt3" <- w33
      "Task" <- T10 ? ("Do Measurement")
    }
  }
  n26 = local read "PI SystemNumber"() -> (w9:i32)
  n27 = control-ref of="X-Position"() -> (w13:refnum<vi>)
  n28 = control-ref of="Y-Position"() -> (w12:refnum<vi>)
  n29 = control-ref of="Z-Position"() -> (w11:refnum<vi>)
  n30 = call "AndorPhysikInstrumenteInitialisiation.vi"("reference"=w13, "error in (no error)"=w14, "reference 3"=w11, "reference 2"=w12, "Pi"=w9) -> ("error out"=w6:errorcluster, "Device List"=w18:T12)  [unwired: 5 in]
  n31 = while {
    shift-right: [w55] -> _
    shift-left: w6 -> [w56]
    stop <- w53 stop-if-true
    n32 = Wait (ms)(milliseconds to wait=u32 ?) -> ()  [unwired: 1 out]
    n33 = local read "Global Stop"() -> (w53:bool)
    n34 = control-ref of="Point"() -> (w52:refnum<vi>)
    n35 = call "RunCameraPreview.vi"("error in (no error)"=w56, "Point 2"=w52) -> ("error out"=w55:errorcluster)  [unwired: 9 in]
  }
  n36 = while {
    tunnel: w6 -> [w73]
    stop <- w59 stop-if-true
    n37 = local read "Global Stop"() -> (w74:bool)
    n38 = local read "Global Stop"() -> (w59:bool)
    n39 = call "Vision Acquisition"("Auto Exposure::Mode"="Auto Exposure::Mode", "Auto Exposure::Value"="Auto Exposure::Value", "Brightness::Mode"="Brightness::Mode", "Brightness::Value"="Brightness::Value", "Gain::Mode"="Gain::Mode", "Stop (F)"=w74, "Gain::Value"="Gain::Value", "error in"=w73, "Gamma::Mode"="Gamma::Mode", "Shutter::Mode"="Shutter::Mode", "Shutter::Value"="Shutter::Value", "Trigger::Trigger Activation"="Trigger::Trigger Activation", "Trigger::Trigger Mode"="Trigger::Trigger Mode", "Trigger::Trigger Parameter"="Trigger::Trigger Parameter", "Trigger Delay::Mode"="Trigger Delay::Mode") -> ("Image Out"=→"Image Out":T5, "Image Number"=→"Image Number":u32, "Frame Rate"=→"acquired FPS":dbl)  [unwired: 8 in, 2 out]
  }
  n40 = while {
    shift-right: [w114] -> _
    shift-left: w6 -> [w116]
    stop <- w115 stop-if-true
    n41 = control-ref of="WS File Tree"() -> (w89:refnum<vi>)
    n42 = local read "Global Stop"() -> (w115:bool)
    n43 = global read "GlobalLaserInterface.vi" "InterfaceLaserInitalised"() -> (w77:refnum<visa-resource-name>)
    n44 = event shown="[19] \"Set Temperature\": Value Change" {
      selector: _ -> [_ _ _ _ _ _ _ _ _ _ _ _ _ _ _ _ _ _ _ _ _ _ _ _ _ _ _ _ _]
      dyn-events: _ -> [_ _ _ _ _ _ _ _ _ _ _ _ _ _ _ _ _ _ _ _ _ _ _ _ _ _ _ _ _]
      timeout: _ -> [_ _ _ _ _ _ _ _ _ _ _ _ _ _ _ _ _ _ _ _ _ _ _ _ _ _ _ _ _]
      tunnel: w116 -> [w117 w119 _ _ w194 _ w237 _ _ _ w280 w333 w336 w372 _ w432 _ w472 w479 w508 _ w518 w527 w538 w540 _ _ _ w547]
      tunnel: [w117 w119 _ _ w195 _ w236 _ _ _ w279 w325 w334 w369 _ w431 _ w471 _ _ _ w516 _ w537 _ _ _ _ w548] -> w114
      tunnel: w89 -> [_ _ _ _ _ _ _ _ _ _ _ _ w338 w373 _ _ _ _ _ _ _ _ _ _ _ _ _ _ _]
      tunnel: "Aquire Image" -> [_ _ _ _ _ _ _ _ _ _ _ _ _ _ _ _ _ _ _ _ _ _ _ _ _ _ _ _ _]
      tunnel: "Save Color Image" -> [_ _ _ _ _ _ _ _ _ _ _ _ _ _ _ _ _ _ _ _ _ _ _ _ _ _ _ _ _]
      tunnel: "Open MSW" -> [_ _ _ _ _ _ _ _ _ _ _ _ _ _ _ _ _ _ _ _ _ _ _ _ _ _ _ _ _]
      tunnel: "Find Mols" -> [_ _ _ _ _ _ _ _ _ _ _ _ _ _ _ _ _ _ _ _ _ _ _ _ _ _ _ _ _]
      tunnel: "Auto Meas" -> [_ _ _ _ _ _ _ _ _ _ _ _ _ _ _ _ _ _ _ _ _ _ _ _ _ _ _ _ _]
      tunnel: "New MSW" -> [_ _ _ _ _ _ _ _ _ _ _ _ _ _ _ _ _ _ _ _ _ _ _ _ _ _ _ _ _]
      tunnel: "Stop Program" -> [_ _ _ _ _ _ _ _ _ _ _ _ _ _ _ _ _ _ _ _ _ _ _ _ _ _ _ _ _]
      tunnel: "Point Measurement" -> [_ _ _ _ _ _ _ _ _ _ _ _ _ _ _ _ _ _ _ _ _ _ _ _ _ _ _ _ _]
      tunnel: "Move Stage" -> [_ _ _ _ _ _ _ _ _ _ _ _ _ _ _ _ _ _ _ _ _ _ _ _ _ _ _ _ _]
      tunnel: w77 -> [_ _ _ _ _ _ _ _ _ _ _ _ _ _ _ _ _ _ _ _ _ _ _ _ _ _ _ _ _]
      tunnel: "Get Position" -> [_ _ _ _ _ _ _ _ _ _ _ _ _ _ _ _ _ _ _ _ _ _ _ _ _ _ _ _ _]
      tunnel: [_ _ _ _ _ _ _ _ _ _ w275 w318 _ _ _ _ _ _ _ _ _ _ _ _ _ _ _ _ _] -> w104
      tunnel: [_ _ _ _ _ _ _ _ _ _ w276 w319 _ _ _ _ _ _ _ _ _ _ _ _ _ _ _ _ _] -> w88
      tunnel: [_ _ _ _ _ _ _ _ _ _ w277 w320 _ _ _ _ _ _ _ _ _ _ _ _ _ _ _ _ _] -> w103
      tunnel: "How long?" -> [_ _ _ _ _ _ _ _ _ _ _ _ _ _ _ _ _ _ _ _ _ _ _ _ _ _ _ _ _]
      tunnel: "Start 3D FCS Abel Scan" -> [_ _ _ _ _ _ _ _ _ _ _ _ _ _ _ _ _ _ _ _ _ _ _ _ _ _ _ _ _]
      tunnel: "Mesaurement Time (Sec) / Step" -> [_ _ _ w153 w199 _ _ _ _ _ _ _ _ _ _ _ _ _ _ _ _ _ _ _ _ _ w545 _ _]
      tunnel: "Y Stepsize" -> [_ _ _ w152 w198 _ _ _ _ _ _ _ _ _ _ _ _ _ _ _ _ _ _ _ _ _ _ _ _]
      tunnel: "X Stepsize" -> [_ _ _ w151 w197 _ _ _ _ _ _ _ _ _ _ _ _ _ _ _ _ _ _ _ _ _ _ _ _]
      tunnel: "Z Stepsize" -> [_ _ _ w150 w196 _ _ _ _ _ _ _ _ _ _ _ _ _ _ _ _ _ _ _ _ _ _ _ _]
      tunnel: "FCS Point Measurement" -> [_ _ _ _ _ _ _ _ _ _ _ _ _ _ _ _ _ _ _ _ _ _ _ _ _ _ _ _ _]
      tunnel: "Z End" -> [_ _ _ w149 w208 _ _ _ _ _ _ _ _ _ _ _ _ _ _ _ _ _ _ _ _ _ _ _ _]
      tunnel: "X End" -> [_ _ _ w148 w202 _ _ _ _ _ _ _ _ _ _ _ _ _ _ _ _ _ _ _ _ _ _ _ _]
      tunnel: "Y End" -> [_ _ _ w147 w205 _ _ _ _ _ _ _ _ _ _ _ _ _ _ _ _ _ _ _ _ _ _ _ _]
      tunnel: "Z Start" -> [_ _ _ w146 w188 _ _ _ _ _ _ _ _ _ _ _ _ _ _ _ _ _ _ _ _ _ _ _ _]
      tunnel: "X Start" -> [_ _ _ w145 w190 _ _ _ _ _ _ _ _ _ _ _ _ _ _ _ _ _ _ _ _ _ _ _ _]
      tunnel: "Y Start" -> [_ _ _ w144 w189 _ _ _ _ _ _ _ _ _ _ _ _ _ _ _ _ _ _ _ _ _ _ _ _]
      tunnel: w89 -> [_ _ _ _ _ _ _ _ _ _ _ _ _ _ _ _ _ _ _ _ _ _ _ _ _ _ _ _ _]
      tunnel: "SET CCD" -> [_ _ _ _ _ _ _ _ _ _ _ _ _ _ _ _ _ _ _ _ _ _ _ _ _ _ _ _ _]
      tunnel: "OPEN SHUTER" -> [_ _ _ _ _ _ _ _ _ _ _ _ _ _ _ _ _ _ _ _ _ w517 _ _ _ _ _ _ _]
      tunnel: "Close" -> [_ _ _ _ _ _ _ _ _ _ _ _ _ _ _ _ _ _ _ _ _ _ w526 _ _ _ _ _ _]
      tunnel: "Stop" -> [_ _ _ _ _ _ _ _ _ _ _ _ _ _ _ _ _ _ _ _ _ _ _ _ _ _ _ _ _]
      tunnel: "Start" -> [_ _ _ _ _ _ _ _ _ _ _ _ _ _ _ _ _ _ _ _ _ _ _ _ _ _ _ _ _]
      tunnel: "Gain" -> [_ _ _ _ _ _ _ _ _ _ _ _ _ _ _ _ _ _ _ _ _ _ _ _ _ _ _ _ _]
      tunnel: "Cam (Defocused)" -> [_ _ _ _ _ _ _ _ _ _ _ _ _ _ _ _ _ _ _ _ w515 _ _ _ _ _ _ _ _]
      tunnel: "Set Temperature" -> [_ _ _ _ _ _ _ _ _ _ _ _ _ _ _ _ _ _ _ _ _ _ _ _ _ _ _ _ _]
      tunnel: "SCANNER EMERGENCY" -> [_ _ _ _ _ _ _ _ _ _ _ _ _ _ _ _ _ _ _ _ _ _ _ _ _ _ _ _ _]
      tunnel: "Get Temperature" -> [_ _ _ _ _ _ _ _ _ _ _ _ _ _ _ _ _ _ _ _ _ _ _ _ _ _ _ _ _]
      event #0 {
        n45 = event-data() -> ()  [unwired: 1 in, 2 out]
      }
      event #1 {
        n46 = event-data() -> ()  [unwired: 1 in, 7 out]
        n47 = local write "Global Stop"(bool ? ("Global Stop")) -> ()
      }
      event #2 {
        n48 = event-data() -> ()  [unwired: 1 in, 7 out]
        n49 = local read "Workspace"() -> (w123:path)
        n50 = local read "Running"() -> (w126:bool)
        n51 = Not(x=w126) -> (.not. x?=w125:bool)
        n52 = Not Equal?(x=w123, y=path ?) -> (x != y?=w121:bool)
        n53 = local read "Task"() -> (w120:T10)
        n54 = case shown="True" w121 {
          tunnel: w125 -> [_ w130]
          tunnel: T13 ? ("Do Measurement") -> [_ w129]
          tunnel: w120 -> [_ w128]
          frame #0 {
            # "No Workspace Open"
            n55 = One Button Dialog(message=string ?) -> ()  [unwired: 1 in, 1 out]
          }
          frame #1 {
            # "Aquire Image if not Running"
            n56 = case shown="True" w130 {
              tunnel: w129 -> [w133 w136]
              tunnel: w128 -> [w131 _]
              frame #0 {
                n57 = Equal?(x=w131, y=w133) -> (x = y?=w132:bool)
                n58 = case shown="False" w132 {
                  frame #0 {
                  }
                  frame #1 {
                    n59 = local write "Stop Measurement"(bool ? ("Stop Measurement")) -> ()
                  }
                }
              }
              frame #1 {
                n60 = local write "Task"(w136) -> ()
                n61 = local write "Running"(bool ? ("Measurement Running")) -> ()
                n62 = property on="Aquire Image" class="Bool"("BoolText.Text"=string ? ("Caption.Text"), "BoolText.TextColor"=u32 ? ("Boolean Text.Colors:FG Color")) -> ()  [unwired: 2 in, 2 out]
              }
            }
          }
        }
      }
      event #3 {
        n63 = event-data() -> ()  [unwired: 1 in, 5 out]
        n64 = Build Array(w153, w152, w151, w150, w149, w148, w147, w146, w145, w144) -> (w143:dbl[])
        n65 = for {
          tunnel: w143 -> [w181] mode=indexing
          tunnel: [w180] -> w142 mode=indexing
          n66 = Not Equal To 0?(x=w181) -> (x != 0?=w180:bool)
        }
        n67 = Boolean Array To Number(Boolean array=w142) -> (number=w141:u32)
        n68 = Not Equal To 0?(x=w141) -> (x != 0?=w140:bool)
        n69 = case shown="True" w140 {
          tunnel: [dbl ? w166] -> w139
          tunnel: w153 -> [_ w165]
          tunnel: w152 -> [_ w164]
          tunnel: w151 -> [_ w163]
          tunnel: w150 -> [_ w162]
          tunnel: w149 -> [_ w161]
          tunnel: w148 -> [_ w160]
          tunnel: w147 -> [_ w159]
          tunnel: w146 -> [_ w158]
          tunnel: w145 -> [_ w157]
          tunnel: w144 -> [_ w156]
          frame #0 {
            n70 = One Button Dialog(message=string ?) -> ()  [unwired: 1 in, 1 out]
          }
          frame #1 {
            w167 = dbl ? ("y")
            # "to hours"
            # "to minutes"
            n71 = Subtract(x=w161, y=w158) -> (x-y=w174:dbl)
            n72 = Subtract(x=w160, y=w157) -> (x-y=w179:dbl)
            n73 = Subtract(x=w159, y=w156) -> (x-y=w176:dbl)
            n74 = Divide(x=w174, y=w162) -> (x/y=w175:dbl)
            n75 = Divide(x=w179, y=w163) -> (x/y=w178:dbl)
            n76 = Divide(x=w176, y=w164) -> (x/y=w177:dbl)
            n77 = Multiply(x=w165, y=w175) -> (x*y=w171:dbl)
            n78 = Multiply(x=w165, y=w178) -> (x*y=w173:dbl)
            n79 = Multiply(x=w165, y=w177) -> (x*y=w172:dbl)
            n80 = Add(x=w173, y=w172) -> (x+y=w170:dbl)
            n81 = Add(x=w171, y=w170) -> (x+y=w169:dbl)
            n82 = Divide(x=w169, y=w167) -> (x/y=w168:dbl)
            n83 = Divide(x=w168, y=w167) -> (x/y=w166:dbl)
          }
        }
        "Estimated Time (h)" <- w139
      }
      event #4 {
        w191 = i32 ?
        n84 = event-data() -> ()  [unwired: 1 in, 5 out]
        n85 = property on="Measurement Time" class="DigNum (strict)"("Value"=w199) -> ()  [unwired: 2 in, 2 out]
        n86 = case shown="No Error" w194 {
          selector: w194 -> [w209 w211]
          tunnel: [w209 w211] -> w183
          frame #0 {
            n87 = global write "StopGetPic.vi" "Stop"(bool ? ("Stop")) -> ()
          }
          frame #1 {
          }
        }
        n88 = local write "Z Stepsize"(w196) -> ()
        n89 = local write "X-Position"(w190) -> ()
        n90 = local write "Y-Position"(w189) -> ()
        n91 = local write "Y Stepsize"(w198) -> ()
        n92 = local write "Z-Position"(w188) -> ()
        n93 = local write "X Stepsize"(w197) -> ()
        n94 = Subtract(x=w202, y=w190) -> (x-y=w201:dbl)
        n95 = Subtract(x=w208, y=w188) -> (x-y=w206:dbl)
        n96 = Subtract(x=w205, y=w189) -> (x-y=w204:dbl)
        n97 = Divide(x=w201, y=w197) -> (x/y=→"X Steps":dbl)
        n98 = Divide(x=w206, y=w196) -> (x/y=→"Z Steps":dbl)
        n99 = Divide(x=w204, y=w198) -> (x/y=→"Y Steps":dbl)
        n100 = local read "PI SystemNumber"() -> (w193:i32)
        n101 = Subtract(x=w191, y=w188) -> (x-y=w185:dbl)
        n102 = Subtract(x=w191, y=w189) -> (x-y=w186:dbl)
        n103 = Subtract(x=w191, y=w190) -> (x-y=w187:dbl)
        n104 = Build Array(w187, w186, w185) -> (w184:dbl[])
        n105 = global read "GlobalConAxisPI.vi" "Conn. Axes"() -> (w192:string[])
        n106 = call "MOV.vi"("System no."=w193, "Axes to move"=w192, "Position values"=w184, "error in"=w183) -> ("error out"=w182:errorcluster)  [unwired: 15 in]
        n107 = case shown="No Error" w182 {
          selector: w182 -> [w212 w214]
          tunnel: [w212 w214] -> w195
          frame #0 {
            "3dAbelFcs" <- bool ?
          }
          frame #1 {
          }
        }
      }
      event #5 {
        n108 = event-data() -> ()  [unwired: 1 in, 7 out]
        n109 = local read "Workspace"() -> (w222:path)
        n110 = local read "Running"() -> (w225:bool)
        n111 = local read "Last Image File No"() -> (w219:i32)
        n112 = Not(x=w225) -> (.not. x?=w224:bool)
        n113 = Not Equal?(x=w222, y=path ?) -> (x != y?=w217:bool)
        n114 = Not Equal?(x=w219, y=i32 ?) -> (x != y?=w216:bool)
        n115 = And(x=w217, y=w216) -> (x .and. y?=w215:bool)
        n116 = local read "Task"() -> (w223:T10)
        n117 = case shown="False" w215 {
          tunnel: w224 -> [_ w229]
          tunnel: T14 ? ("Do Measurement") -> [_ w228]
          tunnel: w223 -> [_ w227]
          frame #0 {
            # "No Workspace Open"
            n118 = One Button Dialog(message=string ?) -> ()  [unwired: 1 in, 1 out]
          }
          frame #1 {
            # "Start Auto Measurement"
            n119 = case shown="True" w229 {
              tunnel: w228 -> [_ w233]
              tunnel: w227 -> [_ _]
              frame #0 {
                n120 = case shown="True" bool ? {
                  frame #0 {
                  }
                  frame #1 {
                    n121 = local write "Stop Measurement"(bool ? ("Stop Measurement")) -> ()
                  }
                }
              }
              frame #1 {
                n122 = local write "Task"(w233) -> ()
                n123 = local write "Running"(bool ? ("Measurement Running")) -> ()
                n124 = local write "NxtAutMesPoint"(i32 ? ("NxtAutMesPoint")) -> ()
              }
            }
          }
        }
      }
      event #6 {
        n125 = event-data() -> ()  [unwired: 1 in, 5 out]
        n126 = call "GetTemperature.vi"("error in (no error)"=w237) -> ("error out"=w238:errorcluster, "temperature"=w241:i32)  [unwired: 3 in, 2 out]
        n127 = call "Build Text"("Cam"=w241, "error in (no error)"=w238) -> ("Result"=w240:string, "error out"=w239:errorcluster)  [unwired: 12 in]
        n128 = call "Display Message to User"("error in (no error)"=w239, "Enable"=bool ?, "Message"=w240) -> ("error out"=w236:errorcluster)  [unwired: 7 in, 1 out]
      }
      event #7 {
        n129 = event-data() -> ()  [unwired: 1 in, 7 out]
        n130 = local read "Active pt3"() -> (w244:path)
        n131 = Not Equal?(x=w244, y=path ?) -> (x != y?=w242:bool)
        n132 = case shown="True" w242 {
          tunnel: T15 ? ("Do Measurement") -> [_ w248]
          frame #0 {
            # "No Workspace Open"
            n133 = One Button Dialog(message=string ?) -> ()  [unwired: 1 in, 1 out]
          }
          frame #1 {
            # "Aquire Image if not Running"
            n134 = local write "Task"(w248) -> ()
            n135 = local write "Running"(bool ? ("Measurement Running")) -> ()
          }
        }
      }
      event #8 {
        n136 = event-data() -> ()  [unwired: 1 in, 7 out]
        n137 = local read "Active pt3"() -> (w251:path)
        n138 = Not Equal?(x=w251, y=path ?) -> (x != y?=w249:bool)
        n139 = case shown="True" w249 {
          tunnel: T15 ? ("Do Measurement") -> [_ w255]
          frame #0 {
            # "No Workspace Open"
            n140 = One Button Dialog(message=string ?) -> ()  [unwired: 1 in, 1 out]
          }
          frame #1 {
            # "Aquire Image if not Running"
            n141 = local write "Task"(w255) -> ()
            n142 = local write "Running"(bool ? ("Measurement Running")) -> ()
          }
        }
      }
      event #9 {
        n143 = event-data() -> ()  [unwired: 1 in, 7 out]
        n144 = local read "Workspace"() -> (w258:path)
        n145 = local read "Running"() -> (w262:bool)
        n146 = Not(x=w262) -> (.not. x?=w261:bool)
        n147 = Not Equal?(x=w258, y=path ?) -> (x != y?=w256:bool)
        n148 = local read "Task"() -> (w259:T10)
        n149 = case shown="True" w256 {
          tunnel: w261 -> [_ w266]
          tunnel: T13 ? ("Do Measurement") -> [_ w265]
          tunnel: w259 -> [_ w264]
          frame #0 {
            # "No Workspace Open"
            n150 = One Button Dialog(message=string ?) -> ()  [unwired: 1 in, 1 out]
          }
          frame #1 {
            # "Aquire Image if not Running"
            n151 = case shown="False" w266 {
              tunnel: w265 -> [w268 w272]
              tunnel: w264 -> [w269 _]
              frame #0 {
                n152 = Equal?(x=w269, y=w268) -> (x = y?=w267:bool)
                n153 = case shown="False" w267 {
                  frame #0 {
                  }
                  frame #1 {
                    n154 = local write "Stop Measurement"(bool ? ("Stop Measurement")) -> ()
                  }
                }
              }
              frame #1 {
                n155 = local write "Task"(w272) -> ()
                n156 = local write "Running"(bool ? ("Measurement Running")) -> ()
                n157 = property on="Point Measurement" class="Bool"("BoolText.Text"=string ? ("Caption.Text"), "BoolText.TextColor"=u32 ? ("Boolean Text.Colors:FG Color")) -> ()  [unwired: 2 in, 2 out]
              }
            }
          }
        }
      }
      event #10 {
        n158 = event-data() -> ()  [unwired: 1 in, 3 out]
        n159 = local read "Workspace"() -> (w283:path)
        n160 = local read "Running"() -> (w285:bool)
        n161 = local read "PI SystemNumber"() -> (w278:i32)
        n162 = Not(x=w285) -> (.not. x?=w284:bool)
        n163 = Not Equal?(x=w283, y=path ?) -> (x != y?=w281:bool)
        n164 = case shown="True" w281 {
          tunnel: w284 -> [_ w293]
          tunnel: w280 -> [_ w292]
          tunnel: [_ w291] -> w279
          tunnel: w278 -> [_ w290]
          tunnel: [_ w289] -> w275
          tunnel: [_ w288] -> w276
          tunnel: [_ w287] -> w277
          frame #0 {
            # "No Workspace Open"
            n165 = One Button Dialog(message=string ?) -> ()  [unwired: 1 in, 1 out]
          }
          frame #1 {
            # "Move Stage if not Running"
            n166 = case shown="True" w293 {
              tunnel: w292 -> [_ w317]
              tunnel: [_ w307] -> w291
              tunnel: w290 -> [_ w315]
              tunnel: [_ w294] -> w289
              tunnel: [_ w295] -> w288
              tunnel: [_ w296] -> w287
              frame #0 {
              }
              frame #1 {
                w299 = i32 ?
                n167 = local read "X-Position"() -> (w302:dbl)
                n168 = local read "Y-Position"() -> (w301:dbl)
                n169 = local read "Z-Position"() -> (w306:dbl)
                n170 = Subtract(x=w299, y=w302) -> (x-y=w303:dbl)
                n171 = Subtract(x=w299, y=w301) -> (x-y=w304:dbl)
                n172 = Subtract(x=w299, y=w306) -> (x-y=w305:dbl)
                n173 = Build Array(w303, w304, w305) -> (w316:dbl[])
                n174 = global read "GlobalConAxisPI.vi" "Conn. Axes"() -> (w314:string[])
                n175 = call "MOV.vi"("System no."=w315, "Axes to move"=w314, "Position values"=w316, "error in"=w317) -> ("error out"=w312:errorcluster)  [unwired: 15 in]
                n176 = call "POS?.vi"("System no."=w315, "Axes to query"=w314, "All axes?"=bool ?, "error in"=w312) -> ("Position"=w311:dbl[], "error out"=w307:errorcluster)  [unwired: 14 in]
                n177 = Index Array(array=w311, index #1=i32 ? ("index"), index #2=i32 ? ("index"), index #3=i32 ? ("index")) -> (element #1=w300:dbl, element #2=w297:dbl, element #3=w298:dbl)
                n178 = Subtract(x=w299, y=w300) -> (x-y=w296:dbl)
                n179 = Subtract(x=w299, y=w297) -> (x-y=w295:dbl)
                n180 = Subtract(x=w299, y=w298) -> (x-y=w294:dbl)
              }
            }
          }
        }
        n181 = property on="y-position" class="DigNum (strict)"("Value"=w276) -> ()  [unwired: 2 in, 2 out]
        n182 = property on="z-position" class="DigNum (strict)"("Value"=w275) -> ()  [unwired: 2 in, 2 out]
        n183 = property on="x-position" class="DigNum (strict)"("Value"=w277) -> ()  [unwired: 2 in, 2 out]
      }
      event #11 {
        w324 = i32 ?
        n184 = event-data() -> ()  [unwired: 1 in, 5 out]
        n185 = local read "PI SystemNumber"() -> (w332:i32)
        n186 = global read "GlobalConAxisPI.vi" "Conn. Axes"() -> (w331:string[])
        n187 = call "POS?.vi"("System no."=w332, "Axes to query"=w331, "All axes?"=bool ?, "error in"=w333) -> ("Position"=w329:dbl[], "error out"=w325:errorcluster)  [unwired: 14 in]
        n188 = Index Array(array=w329, index #1=i32 ? ("index"), index #2=i32 ? ("index"), index #3=i32 ? ("index")) -> (element #1=w321:dbl, element #2=w322:dbl, element #3=w323:dbl)
        n189 = Subtract(x=w324, y=w321) -> (x-y=w320:dbl)
        n190 = Subtract(x=w324, y=w322) -> (x-y=w319:dbl)
        n191 = Subtract(x=w324, y=w323) -> (x-y=w318:dbl)
        n192 = property on="y-position" class="DigNum (strict)"("Value"=w319) -> ()  [unwired: 2 in, 2 out]
        n193 = property on="x-position" class="DigNum (strict)"("Value"=w320) -> ()  [unwired: 2 in, 2 out]
        n194 = property on="z-position" class="DigNum (strict)"("Value"=w318) -> ()  [unwired: 2 in, 2 out]
      }
      event #12 {
        # "Default Name"
        n195 = event-data() -> ()  [unwired: 1 in, 7 out]
        n196 = flat-sequence {
          tunnel: [w354] -> w337
          tunnel: w336 -> [w354]
          frame #0 {
            n197 = local write "Running"(bool ? ("MeasRunig")) -> ()
          }
        }
        n198 = Get Date/Time In Seconds() -> (seconds since 1Jan1904=w351:timestamp)
        n199 = Format Date/Time String(time format string (%c)=string ?, seconds (now)=w351) -> (date/time string=w349:string)  [unwired: 1 out]
        n200 = Concatenate Strings(w349, string ? ("string")) -> (w347:string)
        n201 = call "File Dialog"("start path"=path ?, "prompt"=string ?, "button label"=string ?, "default name"=w347, "error in"=w337, "pattern (all files)"=string ?, "pattern label"=string ?) -> ("selected path"=w341:path, "cancelled"=w342:bool, "error out"=w340:errorcluster)  [unwired: 5 in, 1 out]
        n202 = case shown="False" w342 {
          tunnel: w341 -> [w360 _]
          tunnel: w340 -> [w366 w368]
          tunnel: [w358 w367] -> w335
          tunnel: w338 -> [w356 _]
          frame #0 {
            # "Create Empty Workspace"
            n203 = local write "Workspace"(w360) -> ()
            n204 = call "MTS_CreateWriteMSW.vi"("Rewrite"=bool ?, "error in (no error)"=w366, "Workspace Path"=w360) -> ("error out"=w359:errorcluster, "Created"=w363:string, "Comment (dup)"=w362:string, "Files in Workspace (dup)"=w361:T19)  [unwired: 5 in]
            n205 = call "MTS_Workspace.vi"("Workspace"=w360, "Operation"=T16 ?, "Created in"=w363, "New Comment"=w362, "Files in Workspace in"=w361) -> ("Files in Workspace"=w357:T20)  [unwired: 3 in, 3 out]
            n206 = call "MTS_BuildWSTree.vi"("error in"=w359, "Files in Workspace"=w357, "Tree Refnum"=w356) -> ("error out"=w358:errorcluster)  [unwired: 6 in, 2 out]
          }
          frame #1 {
            n207 = call <vilib>:"Clear Errors.vi"("error in (no error)"=w368) -> ("error out"=w367:errorcluster)  [unwired: 6 in]
          }
        }
        n208 = flat-sequence {
          tunnel: w335 -> [w352]
          tunnel: [w352] -> w334
          frame #0 {
            n209 = local write "Running"(bool ? ("MeasRunig")) -> ()
          }
        }
      }
      event #13 {
        n210 = event-data() -> ()  [unwired: 1 in, 7 out]
        n211 = flat-sequence {
          tunnel: w372 -> [w384]
          tunnel: [w384] -> w371
          frame #0 {
            n212 = local write "Running"(bool ? ("MeasRunig")) -> ()
          }
        }
        n213 = call "File Dialog2"("start path"=path ?, "prompt"=string ?, "button label"=string ?, "error in"=w371, "pattern (all files)"=string ?, "pattern label"=string ?) -> ("selected path"=w376:path, "cancelled"=w377:bool, "error out"=w375:errorcluster)  [unwired: 6 in, 1 out]
        n214 = case shown="False" w377 {
          tunnel: w376 -> [w392 _]
          tunnel: w375 -> [w397 w399]
          tunnel: [w390 w398] -> w370
          tunnel: w373 -> [w389 _]
          frame #0 {
            # "Open Workspace"
            n215 = local write "Workspace"(w392) -> ()
            n216 = call "MTS_ReadMSW.vi"("error in (no error)"=w397, "Workspace Path"=w392) -> ("error out"=w391:errorcluster, "Created"=w395:string, "Comment"=w394:string, "Files in Workspace"=w393:T21)  [unwired: 6 in]
            n217 = call "MTS_Workspace.vi"("Workspace"=w392, "Operation"=T16 ?, "Created in"=w395, "New Comment"=w394, "Files in Workspace in"=w393) -> ("Files in Workspace"=w388:T20)  [unwired: 3 in, 3 out]
            n218 = Array To Cluster(array=w388) -> (cluster=w387:T22)
            n219 = Unbundle By Name(w387) -> ()  [unwired: 1 out]
            n220 = call "MTS_BuildWSTree.vi"("error in"=w391, "Files in Workspace"=w388, "Tree Refnum"=w389) -> ("error out"=w390:errorcluster, "numberOfFilesInWorkspace"=w386:i32)  [unwired: 6 in, 1 out]
            n221 = local write "Last Image File No"(w386) -> ()
          }
          frame #1 {
            n222 = call <vilib>:"Clear Errors.vi"("error in (no error)"=w399) -> ("error out"=w398:errorcluster)  [unwired: 6 in]
          }
        }
        n223 = flat-sequence {
          tunnel: w370 -> [w382]
          tunnel: [w382] -> w369
          frame #0 {
            n224 = local write "Running"(bool ? ("MeasRunig")) -> ()
          }
        }
      }
      event #14 {
        w402 = dbl ? ("y")
        n225 = event-data() -> ("Coords"=w414:T23, "PlatMods"=w415:T24)  [unwired: 1 in, 5 out]
        n226 = invoke on="Image" class="IntGraph (strict)" method="Map Coords To XY"("Coords"=w414) -> ("Map Coords To XY"=w411:bool, "XY"=w409:cluster{"X":dbl, "Y":dbl})  [unwired: 6 in, 5 out]
        n227 = Unbundle By Name(w415) -> ("Ctrl"=w412:bool)
        n228 = And(x=w411, y=w412) -> (x .and. y?=w413:bool)
        n229 = Unbundle(w409) -> ("X"=w408:dbl, "Y"=w405:dbl)
        n230 = Multiply(x=w408, y=w402) -> (x*y=w407:dbl)
        n231 = Multiply(x=w405, y=w402) -> (x*y=w404:dbl)
        n232 = Round To Nearest(number=w407) -> (nearest integer value=w406:dbl)
        n233 = Round To Nearest(number=w404) -> (nearest integer value=w403:dbl)
        n234 = Divide(x=w406, y=w402) -> (x/y=w401:dbl)
        n235 = Divide(x=w403, y=w402) -> (x/y=w400:dbl)
        n236 = local read "Axis"() -> (w410:enum32{"x-y", "x-z", "y-x", "y-z", "z-x", "z-y"})
        n237 = case shown="True" w413 {
          tunnel: w410 -> [_ w418]
          tunnel: w401 -> [_ w417]
          tunnel: w400 -> [_ w416]
          frame #0 {
          }
          frame #1 {
            n238 = case shown="\"x-y\", Default" w418 {
              tunnel: w417 -> [w420 w422 w424]
              tunnel: w416 -> [w419 w421 w423]
              frame #0 {
                n239 = local write "X-Position"(w420) -> ()
                n240 = local write "Y-Position"(w419) -> ()
              }
              frame #1 {
                n241 = local write "X-Position"(w422) -> ()
                n242 = local write "Z-Position"(w421) -> ()
              }
              frame #2 {
                n243 = local write "Y-Position"(w424) -> ()
                n244 = local write "Z-Position"(w423) -> ()
              }
            }
          }
        }
      }
      event #15 {
        n245 = event-data() -> ("NewVal"=w433:string)  [unwired: 1 in, 4 out]
        n246 = control-ref of="Workspace"() -> (w430:refnum<vi>)
        n247 = control-ref of="Histogram"() -> (w428:refnum<vi>)
        n248 = control-ref of="Trace"() -> (w427:refnum<vi>)
        n249 = control-ref of="Image"() -> (w426:refnum<vi>)
        n250 = control-ref of="Image"() -> (w425:refnum<vi>)
        n251 = control-ref of="Active pt3"() -> (w429:refnum<vi>)
        n252 = call "CreateNewWSfile.vi"("reference 5"=w425, "NewVal"=w433, "Image"=w426, "reference in"=w429, "error in (no error)"=w432, "reference 4"=w427, "reference 3"=w428, "Path in"=w430) -> ("error out"=w431:errorcluster)  [unwired: 3 in]
      }
      event #16 {
        n253 = event-data() -> ()  [unwired: 1 in, 5 out]
        n254 = local read "Axis"() -> (w454:enum32{"x-y", "x-z", "y-x", "y-z", "z-x", "z-y"})
        n255 = local read "Picture size"() -> (w456:dbl)
        n256 = local read "X-Position"() -> (w451:dbl)
        n257 = local read "Y-Position"() -> (w450:dbl)
        n258 = local read "Z-Position"() -> (w449:dbl)
        n259 = local read "Resolution"() -> (w448:dbl)
        n260 = local read "Pixel time"() -> (w457:dbl)
        n261 = local write "Axis"(w454) -> ()
        n262 = local read "Picture size 2"() -> (w455:dbl)
        n263 = local read "Laser  Profile"() -> (w438:string)
        n264 = local write "Pixel time"(w457) -> ()
        n265 = call "PI_CheckScan.vi"("Picture size"=w456, "Picture size 2"=w455, "Axis"=w454, "x-Position"=w451, "y-Position"=w450, "z-Position"=w449) -> ("Picture size out"=w452:dbl, "Picture size out 2"=w453:dbl)  [unwired: 8 in, 4 out]
        n266 = String To Byte Array(string=w438) -> (unsigned byte array=w436:u8[])
        n267 = Divide(x=w452, y=w448) -> (x/y=w460:dbl)
        n268 = local write "Picture size"(w452) -> ()
        n269 = Divide(x=w453, y=w448) -> (x/y=w461:dbl)
        n270 = local write "Picture size 2"(w453) -> ()
        n271 = Array Size(array=w436) -> (size(s)=w435:i32)
        n272 = Subtract(x=w436, y=i32 ?) -> (x-y=w442:i32[])
        n273 = Round Toward +Infinity(x=w460) -> (ceil(x): smallest int >= x=→"x":dbl)
        n274 = Round Toward +Infinity(x=w461) -> (ceil(x): smallest int >= x=→"y":dbl)
        n275 = Initialize Array(i32 ?, w435) -> (w446:i32[])
        n276 = Initialize Array(i32 ?, w435) -> (w444:i32[])
        n277 = In Range and Coerce(upper limit=w446, x=w442, lower limit=w444) -> (coerced(x)=w439:i32[])  [unwired: 1 out]
        n278 = Add(x=w439, y=i32 ?) -> (x+y=w441:i32[])
        n279 = Byte Array To String(unsigned byte array=w441) -> (string=w437:string)
        n280 = while {
          shift-right: [w466] -> w434
          shift-left: w437 -> [w470]
          i -> [w462]
          stop <- w465 stop-if-true
          n281 = Increment(x=w462) -> (x+1=w463:i32)
          n282 = String Subset(string=w470, offset (0)=w462, length (rest)=i32 ?) -> (substring=w468:string)
          n283 = Search and Replace String(replace all?=bool ?, input string=w470, search string=w468, offset=w463) -> (result string=w466:string)  [unwired: 4 in, 3 out]
          n284 = String Length(string=w466) -> (length=w464:i32)
          n285 = Less?(x=w464, y=w462) -> (x < y?=w465:bool)
        }
        n286 = local write "Laser  Profile"(w434) -> ()
      }
      event #17 {
        n287 = event-data() -> ()  [unwired: 1 in, 5 out]
        n288 = local read "PI SystemNumber"() -> (w473:i32)
        n289 = call "PI Write GPIB.vi"("System no."=w473, "String to send"=string ?, "error in"=w472) -> ("error out"=w475:errorcluster)  [unwired: 16 in]
        n290 = flat-sequence {
          tunnel: [w476] -> w471
          tunnel: w475 -> [w476]
          frame #0 {
            n291 = One Button Dialog(message=string ?) -> ()  [unwired: 2 out]
          }
        }
      }
      event #18 {
        n292 = event-data() -> ()  [unwired: 1 in, 6 out]
        n293 = call "Camera CCD Chip settings"("error in (no error)"=w479) -> ("Horizontal Binning"=w480:dbl, "Vertical Binning"=w485:dbl, "CCD Chip Horizontal Start"=w484:dbl, "CCD Chip Horizontal End"=w482:dbl, "CCD Chip Vertical Start"=w483:dbl, "CCD Chip Vertical End"=w481:dbl, "OK"=w486:bool, "error out"=w478:errorcluster)  [unwired: 11 in]
        n294 = case shown="True" w486 {
          tunnel: w485 -> [_ w494]
          tunnel: w484 -> [_ w493]
          tunnel: w483 -> [_ w492]
          tunnel: w482 -> [_ w491]
          tunnel: w481 -> [_ w490]
          tunnel: w480 -> [_ w489]
          tunnel: [_ w488] -> _
          tunnel: w478 -> [_ w487]
          frame #0 {
          }
          frame #1 {
            n295 = flat-sequence {
              tunnel: w494 -> [w501]
              tunnel: w493 -> [w495]
              tunnel: w492 -> [w500]
              tunnel: w491 -> [w499]
              tunnel: w490 -> [w498]
              tunnel: w489 -> [w497]
              tunnel: [w496] -> w488
              tunnel: w487 -> [w496]
              frame #0 {
                n296 = global write "GlobalSetGetConfigureCamera.vi" "Vbin"(w501) -> ()
                n297 = global write "GlobalSetGetConfigureCamera.vi" "Hbin"(w497) -> ()
                n298 = global write "ccdChipPixels.vi" "CCD Chip horizontal start"(w495) -> ()
                n299 = global write "ccdChipPixels.vi" "CCD Chip Vertical Start"(w500) -> ()
                n300 = global write "ccdChipPixels.vi" "CCD Chip horizontal end"(w499) -> ()
                n301 = global write "ccdChipPixels.vi" "CCD Chip Vertical end"(w498) -> ()
                n302 = Subtract(x=w499, y=w495) -> (x-y=w503:dbl)
                n303 = Subtract(x=w498, y=w500) -> (x-y=w502:dbl)
                n304 = Increment(x=w503) -> (x+1=w505:dbl)
                n305 = Increment(x=w502) -> (x+1=w504:dbl)
                n306 = Multiply(x=w505, y=w504) -> (x*y=w506:dbl)
                n307 = global write "ccdChipPixels.vi" "CCD Chip Size"(w506) -> ()
              }
            }
          }
        }
      }
      event #19 {
        n308 = event-data() -> ()  [unwired: 1 in, 6 out]
        n309 = call "camera cooling"("error in (no error)"=w508) -> ("Temperature"=w509:dbl, "OK"=w510:bool, "error out"=w507:errorcluster)  [unwired: 16 in]
        n310 = case shown="True" w510 {
          tunnel: w509 -> [_ w514]
          tunnel: w507 -> [w511 w513]
          tunnel: [w511 w512] -> _
          frame #0 {
          }
          frame #1 {
            n311 = call "CheckTemperature.vi"("error in (no error)"=w513, "temperature in"=w514) -> ("error out"=w512:errorcluster)  [unwired: 9 in]
          }
        }
      }
      event #20 {
        n312 = event-data() -> ()  [unwired: 1 in, 6 out]
        n313 = global write "CamDef.vi" "CamDef"(w515) -> ()
      }
      event #21 {
        n314 = event-data() -> ()  [unwired: 1 in, 6 out]
        n315 = case shown="False" w517 {
          tunnel: [T18 ? ("mode") T18 ? ("mode")] -> w521
          tunnel: w518 -> [w523 w524]
          tunnel: [w523 w524] -> w520
          frame #0 {
          }
          frame #1 {
          }
        }
        n316 = call "SetShutter.vi"("type"=T17 ?, "mode"=w521, "error in (no error)"=w520) -> ("error out"=w516:errorcluster)  [unwired: 11 in, 1 out]
      }
      event #22 {
        n317 = event-data() -> ()  [unwired: 1 in, 6 out]
        n318 = case shown="True" w526 {
          tunnel: [T18 ? ("mode") T18 ? ("mode")] -> w530
          tunnel: w527 -> [w532 w533]
          tunnel: [w532 w533] -> w529
          frame #0 {
          }
          frame #1 {
          }
        }
        n319 = call "SetShutter.vi"("type"=T17 ?, "mode"=w530, "error in (no error)"=w529) -> ()  [unwired: 11 in, 2 out]
      }
      event #23 {
        n320 = event-data() -> ()  [unwired: 1 in, 6 out]
        n321 = call "Camera kinetic settings"("error in (no error)"=w538) -> ("Exposure time"=w535:dbl, "OK"=w536:bool, "error out"=w537:errorcluster)  [unwired: 16 in]
        n322 = case shown="True" w536 {
          tunnel: w535 -> [_ w539]
          frame #0 {
          }
          frame #1 {
            n323 = global write "GlobalSetGetConfigureCamera.vi" "Exposure"(w539) -> ()
          }
        }
      }
      event #24 {
        n324 = event-data() -> ()  [unwired: 1 in, 6 out]
        n325 = call "set gain"("error in (no error)"=w540) -> ("gain"=w542:dbl, "OK"=w541:bool)  [unwired: 16 in, 1 out]
        n326 = case shown="True" w541 {
          tunnel: w542 -> [_ w543]
          frame #0 {
          }
          frame #1 {
            n327 = global write "GlobalSetGetConfigureCamera.vi" "gain"(w543) -> ()
          }
        }
      }
      event #25 {
        n328 = event-data() -> ()  [unwired: 1 in, 6 out]
        n329 = global write "GetPicture.vi" "GetPicture"(bool ? ("GetPicture")) -> ()
      }
      event #26 {
        n330 = event-data() -> ()  [unwired: 1 in, 6 out]
        n331 = global write "GlobalSetGetConfigureCamera.vi" "Exposure"(w545) -> ()
      }
      event #27 {
        n332 = event-data() -> ()  [unwired: 1 in, 6 out]
        n333 = global write "StopGetPic.vi" "Stop"(bool ? ("Stop")) -> ()
      }
      event #28 {
        n334 = event-data() -> ()  [unwired: 1 in, 6 out]
        n335 = flat-sequence {
          tunnel: w547 -> [w551]
          tunnel: [w551] -> w550
          frame #0 {
            n336 = local write "Global Stop"(bool ? ("Global Stop")) -> ()
          }
        }
        n337 = local read "PI SystemNumber"() -> (w549:i32)
        n338 = call "Close connection if open.vi"("System no."=w549, "error in"=w550) -> ("error out"=w548:errorcluster)  [unwired: 16 in, 1 out]
      }
    }
    "z-position" <- w104
    "y-position" <- w88
    "x-position" <- w103
  }
  n339 = while {
    shift-right: [w559] -> w10
    shift-left: w6 -> [w556]
    shift-right: [w561] -> _
    shift-left: w6 -> [w566]
    tunnel: w18 -> [w560]
    tunnel: "Image Measurent Parameters" -> [w555]
    tunnel: [w554] -> _
    tunnel: "Sample description" -> [w553]
    stop <- w564 stop-if-true
    n340 = case shown="No Error" w556 {
      selector: w556 -> [w572 w1447]
      tunnel: w566 -> [w582 w1449]
      tunnel: [w581 bool ? ("Global Stop")] -> w563
      tunnel: [w577 w1449] -> w562
      tunnel: w560 -> [w576 _]
      tunnel: [w575 w1447] -> w559
      tunnel: [w573 T25 ? ("Do Measurement")] -> w557
      tunnel: w555 -> [w570 _]
      tunnel: [w569 w1447] -> w554
      tunnel: w553 -> [w567 _]
      frame #0 {
        n341 = while {
          shift-right: [w1445] -> w578
          shift-left: w582 -> [w1445]
          tunnel: [w1440] -> w580
          tunnel: [w1442] -> w579
          tunnel: [w1441] -> w574
          stop <- w1446 stop-if-true
          w1441 = bool ? ("FiFo Overrun")
          # "Wait for Start"
          n342 = local read "Task"() -> (w1440:T10)
          n343 = local read "Global Stop"() -> (w1442:bool)
          n344 = Wait (ms)(milliseconds to wait=u32 ?) -> ()  [unwired: 1 out]
          n345 = Greater Than 0?(x=w1440) -> (x > 0?=w1444:bool)
          n346 = local write "Stop Measurement"(w1441) -> ()
          n347 = Or(x=w1444, y=w1442) -> (x .or. y?=w1446:bool)
        }
        n348 = control-ref of="WS File Tree"() -> (w571:refnum<vi>)
        n349 = case shown="\"Find Single Mol.\"" w580 {
          selector: w580 -> [_ _ w949 _ _ _]
          tunnel: w572 -> [w583 w631 w857 w1132 w1201 w1403]
          tunnel: [w583 w601 w905 w1121 w1199 w1403] -> w575
          tunnel: [w584 bool ? ("Global Stop") bool ? ("Global Stop") bool ? ("Global Stop") bool ? ("Global Stop") bool ? ("Global Stop")] -> w581
          tunnel: w579 -> [w584 _ _ _ _ _]
          tunnel: w578 -> [w586 w615 w856 w1131 w1200 w1404]
          tunnel: [w586 w615 w970 w1131 w1200 w1402] -> w577
          tunnel: w576 -> [_ w681 w907 _ _ _]
          tunnel: [T25 ? ("Do Measurement") T25 ? ("Do Measurement") w948 T25 ? ("Do Measurement") T14 ? ("Do Measurement") w1401] -> w573
          tunnel: w571 -> [_ _ w938 _ _ _]
          tunnel: w570 -> [_ w659 _ _ _ _]
          tunnel: [w583 w633 w931 w1121 _ _] -> w569
          tunnel: "Laser pulse duration" -> [_ _ w913 _ _ _]
          tunnel: w567 -> [_ _ w904 _ _ _]
          frame #0 {
          }
          frame #1 {
            w594 = i32 ?
            w625 = T33 ? ("Measurement Type")
            w662 = i32 ? ("dimension size")
            # "TODO:\n- FIFO Read Flag Buffer Half Full?\n- auto square pixels"
            # "Image Intensity Array"
            n350 = Index Array(array=w681) -> (element=w680:T34)  [unwired: 1 in]
            n351 = Unbundle By Name(w680) -> ("Dev"=w653:i32)
            n352 = local read "PI SystemNumber"() -> (w603:i32)
            n353 = Index Array(array=string[] ? ("Array"), index="Axis") -> (element=w608:string)
            n354 = stacked-sequence {
              seq-local: [w693 _] -> [_ w720]
              seq-local: [w692 _] -> [_ w721]
              seq-local: [w691 _] -> [_ w716]
              seq-local: [w687 _] -> [_ w714]
              seq-local: [w686 _] -> [_ w713]
              seq-local: [w685 _] -> [_ w712]
              seq-local: [w688 _] -> [_ w708]
              tunnel: "Picture size" -> [w706 _]
              tunnel: "Picture size 2" -> [w705 _]
              tunnel: w659 -> [w704 _]
              tunnel: "X-Position" -> [w703 _]
              tunnel: "Y-Position" -> [w702 _]
              tunnel: "Z-Position" -> [w701 _]
              tunnel: "Axis" -> [w695 _]
              tunnel: "Resolution" -> [w691 _]
              tunnel: [w694 _] -> w587
              tunnel: [_ w722] -> w632
              tunnel: w631 -> [w689 _]
              tunnel: w608 -> [_ w719]
              tunnel: "Laser  Profile" -> [_ w718]
              tunnel: "Pixel time" -> [w690 w717]
              tunnel: w603 -> [_ w715]
              tunnel: [_ w707] -> w628
              tunnel: [_ w711] -> w627
              tunnel: [_ w710] -> w626
              tunnel: [_ w709] -> w618
              frame #0 {
                n355 = call "PI_CheckScan.vi"("Picture size"=w706, "Picture size 2"=w705, "Axis"=w695, "x-Position"=w703, "y-Position"=w702, "z-Position"=w701, "error in (no error)"=w689) -> ("error out"=w688:errorcluster, "Picture size out"=w692:dbl, "Picture size out 2"=w693:dbl, "a0"=w687:dbl, "b0"=w686:dbl, "c0"=w685:dbl)  [unwired: 7 in]
                n356 = Divide(x=w692, y=w691) -> (x/y=w698:dbl)
                n357 = Divide(x=w693, y=w691) -> (x/y=w699:dbl)
                n358 = local write "Picture size 2"(w693) -> ()
                n359 = local write "Picture size"(w692) -> ()
                n360 = Round Toward +Infinity(x=w698) -> (ceil(x): smallest int >= x=w697:dbl)
                n361 = Round Toward +Infinity(x=w699) -> (ceil(x): smallest int >= x=w696:dbl)
                n362 = Bundle("a0"=w687, "b0"=w686, "c0"=w685) -> (w700:cluster{"a0":dbl, "b0":dbl, "c0":dbl})  [unwired: 1 in]
                n363 = Bundle By Name(cluster=w704, "Position"=w700, "Axis 1 Pixels"=w697, "Axis 2 Pixels"=w696, "Axis"=w695, "Resolution"=w691, "PixelTime"=w690) -> (w694:T8)
              }
              frame #1 {
                n364 = call "PI_AreaScan_Prepare_1.vi"("System"=w715, "Laser"=w718, "Axis"=w719, "da"=w721, "db"=w720, "error in (no error)"=w708, "a0"=w714, "b0"=w713, "Resolution"=w716, "c0"=w712, "Pixel time"=w717) -> ("Tacq"=w707:dbl, "lp"=w710:i32, "ap"=w711:i32, "Trigger"=w709:dbl[], "error out"=w722:errorcluster)  [unwired: 4 in]
                "Measure. time" <- w707
              }
            }
            n365 = String To Byte Array(string="Laser  Profile") -> (unsigned byte array=w610:u8[])
            n366 = Unbundle By Name(w587) -> ("Axis 1 Pixels"=w640:dbl, "Axis 2 Pixels"=w641:dbl, "Resolution"=w638:dbl, "PixelTime"=w622:dbl)  [unwired: 2 out]
            n367 = control-ref of="WS File Tree"() -> (w665:refnum<vi>)
            n368 = local read "Workspace"() -> (w670:path)
            n369 = Divide(x=w640, y=w638) -> (x/y=w649:dbl)
            n370 = Divide(x=w641, y=w638) -> (x/y=w651:dbl)
            n371 = call "HH_Set.vi"("Device List"=w681, "CFD Settings"="CFD Settings", "error in (no error)"=w632, "SyncDiv"=i32 ?) -> ("ht3 header out"=w645:T35, "Sync Rate"=w643:i32, "error out"=w617:errorcluster)  [unwired: 7 in, 2 out]
            n372 = Divide(x=w622, y=i32 ?) -> (x/y=w620:dbl)
            n373 = control-ref of="Image"() -> (w647:refnum<vi>)
            n374 = Round Toward +Infinity(x=w649) -> (ceil(x): smallest int >= x=w648:dbl)
            n375 = Round Toward +Infinity(x=w651) -> (ceil(x): smallest int >= x=w650:dbl)
            n376 = call "MTS_PreapareImage.vi"("WS File Tree"=w665, "Workspace"=w670, "Measurement Type"=w625, "Image Measurent Parameters"=w587, "error in"=w617, "Trigger"=w618) -> ("File Name (dup)"=w655:path, "File No"=→"Last Image File No":i32, "Image Header"=w657:T36, "Comment"=w658:string, "error out"=w616:errorcluster)  [unwired: 5 in]
            n377 = Divide(x=i32 ?, y=w643) -> (x/y=w624:dbl)
            n378 = local write "Active pt3"(w655) -> ()
            n379 = Multiply(x=w628, y=i32 ?) -> (x*y=w637:dbl)
            n380 = call "Scan_SetGraphScales.vi"("error in (no error)"=w616, "Image Measurent Parameters"=w587, "Image"=w647) -> ("error out"=w646:errorcluster)  [unwired: 8 in]
            n381 = Subtract(x=w610, y=i32 ?) -> (x-y=w609:i32[])
            n382 = Initialize Array(i32 ? ("element"), w648, w650) -> (w621:i32[][])
            n383 = Initialize Array(i32 ?, i32 ?, i32 ?) -> (w607:i32[][])
            n384 = Replace Array Subset(array=w607, new element=w609, index (col)=i32 ?) -> (w605:i32[][])  [unwired: 1 in]
            n385 = call "HT3_Create.vi"("Laser"=w605, "Image Header in"=w657, "Save pt3"="Save Files", "Measurement Type"=w625, "error in"=w646, "Comment"=w658, "ht3 Header in"=w645, "File Path"=w655) -> ("error out"=w671:errorcluster, "FileHeaderPos"=w661:T37, "refnum out"=w669:refnum<file>)  [unwired: 1 in]
            n386 = Round Toward +Infinity(x=w637) -> (ceil(x): smallest int >= x=w635:dbl)
            n387 = call "HH_Start.vi"("Device Index"=w653, "Acq. Time"=w635, "error in (no error)"=w671) -> ("error out"=w678:errorcluster)  [unwired: 11 in, 1 out]
            n388 = Unbundle By Name(w678) -> ("status"=w679:bool)
            n389 = Not(x=w679) -> (.not. x?=w677:bool)
            n390 = Initialize Array(u32 ?, w662) -> (w674:u32[])
            n391 = case shown="True" w677 {
              tunnel: [w770 w801] -> w676
              tunnel: w603 -> [_ w796]
              tunnel: w678 -> [w771 w797]
              tunnel: w653 -> [w769 w788]
              tunnel: w621 -> [_ w773]
              tunnel: w674 -> [_ w795]
              tunnel: w662 -> [_ w794]
              tunnel: [w768 w793] -> w673
              tunnel: [w768 w792] -> w672
              tunnel: w669 -> [w767 w791]
              tunnel: [w767 w790] -> w668
              tunnel: [i32 ? ("Num Records Total") w789] -> w667
              tunnel: [dbl ? w782] -> w666
              tunnel: w608 -> [_ w785]
              tunnel: [dbl[] ? w779] -> w623
              tunnel: w620 -> [_ w775]
              tunnel: w618 -> [_ w774]
              frame #0 {
                (unwired) i32[][] ? ("Image Array Out")
                (unwired) u64[] ? ("Histograms")
                w768 = bool ? ("Stop Measurement")
                n392 = call "HH_Stop.vi"("Device Index"=w769, "error in (no error)"=w771) -> ("error out"=w770:errorcluster)  [unwired: 12 in, 1 out]
              }
              frame #1 {
                # "Overflow Interv. Time (s)"
                # "No Error"
                n393 = call "PI Start WG.vi"("System no."=w796, "axis"=w785, "Generator"=T26 ?, "Init DDL"=T27 ?, "increment"=T27 ?, "error in"=w797, "saved data"=T28 ?) -> ("error out"=w798:errorcluster)  [unwired: 12 in]
                n394 = Initialize Array(i32 ?, i32 ?) -> (w776:i32[])
                n395 = while {
                  tunnel: w788 -> [w821]
                  tunnel: w795 -> [w837]
                  tunnel: w794 -> [w836]
                  shift-right: [w822] -> w800
                  shift-left: w798 -> [w838]
                  shift-right: [bool ? ("Reset")] -> _
                  shift-left: bool ? ("Reset") -> [w809]
                  tunnel: [w830] -> w793
                  tunnel: [w826] -> w792
                  tunnel: w791 -> [w828]
                  tunnel: [w827] -> w790
                  tunnel: [w805] -> w789
                  tunnel: [w804] -> w782
                  shift-right: [w818] -> w781
                  shift-left: w776 -> [w816]
                  tunnel: [w815] -> w780
                  tunnel: w775 -> [w812]
                  tunnel: w774 -> [_]
                  shift-right: [w803] -> w772
                  shift-left: w773 -> [w811]
                  i -> [w814]
                  stop <- w835 stop-if-true
                  n396 = call "HH_FIFORead.vi"("Device Index"=w821, "Buffer In"=w837, "Count"=w836, "error in (no error)"=w838) -> ("OK"=w831:bool, "Buffer Out"=w808:u32[], "Data Count"=w807:i32, "FiFo Overrun"=w830:bool, "error out"=w829:errorcluster)  [unwired: 7 in]
                  n397 = Unbundle(w829) -> ("status"=w834:bool)  [unwired: 2 out]
                  n398 = local write "Buffer Overrun"(w830) -> ()
                  n399 = call "HT3_Write.vi"("error in"=w829, "Data Count"=w807, "Data in"=w808, "refnum in"=w828) -> ("error out"=w823:errorcluster, "refnum out"=w827:refnum<file>)  [unwired: 6 in]
                  n400 = call "GetCountRates.vi"("error in (no error)"=w823, "DeviceIndex"=w821) -> ("error out"=w822:errorcluster, "CntRates"=w820:dbl[], "SyncRate"=w813:i32)  [unwired: 1 in]
                  n401 = local read "Stop Measurement"() -> (w825:bool)
                  n402 = local read "Global Stop"() -> (w824:bool)
                  n403 = Multiply(x=w812, y=w813) -> (x*y=w802:dbl)
                  n404 = Compound Arithmetic op=OR(invert w831, w834, w824, w825) -> (w835:bool)
                  n405 = Insert Into Array(array=w820, index=i32 ?, new element=w813) -> (w817:dbl[])
                  n406 = call "HH_ToImage.vi"("Data In"=w808, "Reset"=w809, "Image Array In"=w811, "Data Count"=w807, "Pixel Time (Laser Pulses)"=w802) -> ("Image Array Out"=w803:i32[][], "Histograms"=→"Histogram":i32[][], "Total Oveflow Count"=w804:u64, "Num Records Total"=w805:i64, "Traces"=→"Trace":i32[][])  [unwired: 4 in, 2 out]
                  n407 = Or(x=w825, y=w824) -> (x .or. y?=w826:bool)
                  n408 = Add(x=w816, y=w817) -> (x+y=w818:dbl[])
                  n409 = Wait (ms)(milliseconds to wait=u32 ?) -> ()  [unwired: 1 out]
                  n410 = Increment(x=w814) -> (x+1=w815:i32)
                }
                "Image" <- w772
                n411 = call "HH_Stop.vi"("Device Index"=w788, "error in (no error)"=w800) -> ("error out"=w801:errorcluster)  [unwired: 12 in, 1 out]
                n412 = Divide(x=w781, y=w780) -> (x/y=w779:dbl[])
              }
            }
            n413 = flat-sequence {
              tunnel: w676 -> [w741]
              tunnel: [w730] -> w602
              tunnel: w673 -> [w743]
              tunnel: w672 -> [w732]
              tunnel: w603 -> [w740]
              tunnel: [w739] -> w600
              tunnel: w668 -> [w737]
              tunnel: w667 -> [w736]
              tunnel: w666 -> [w726]
              tunnel: w661 -> [w731]
              tunnel: w624 -> [w727]
              tunnel: w623 -> [w723]
              frame #0 {
                # "Count Rate (per s)"
                # "Finish after Aquire Image"
                n414 = Multiply(x=w727, y=w726) -> (x*y=w725:dbl)
                n415 = Or(x=w732, y=w743) -> (x .or. y?=w742:bool)
                n416 = case shown="False" w742 {
                  tunnel: w741 -> [w748 w758]
                  tunnel: w740 -> [w746 w759]
                  tunnel: [w745 w759] -> w739
                  tunnel: [w747 w757] -> w738
                  tunnel: [enum16{"timeover", "manual", "overflow"} ? ("Stop Reason") w762] -> w733
                  tunnel: w732 -> [w744 w760]
                  frame #0 {
                    # "Stop WaveGen\nif Aborted"
                    n417 = case shown="True" w744 {
                      tunnel: w748 -> [w750 w755]
                      tunnel: [w750 w754] -> w747
                      tunnel: w746 -> [w751 w753]
                      tunnel: [w751 w753] -> w745
                      frame #0 {
                      }
                      frame #1 {
                        n418 = call "PI Write GPIB.vi"("System no."=w753, "String to send"=string ?, "error in"=w755) -> ("error out"=w754:errorcluster)  [unwired: 16 in]
                      }
                    }
                  }
                  frame #1 {
                    n419 = Select(t=enum16{"timeover", "manual", "overflow"} ? ("Stop Reason"), s=w760, f=enum16{"timeover", "manual", "overflow"} ? ("Stop Reason")) -> (s? t:f=w762:enum16{"timeover", "manual", "overflow"})
                    n420 = call "PI Write GPIB.vi"("System no."=w759, "String to send"=string ?, "error in"=w758) -> ("error out"=w757:errorcluster)  [unwired: 16 in]
                  }
                }
                n421 = Multiply(x=w725, y=dbl ?) -> (x*y=w735:dbl)
                n422 = property on="Aquire Image" class="Bool"("BoolText.Text"=string ? ("Caption.Text"), "BoolText.TextColor"=u32 ? ("Boolean Text.Colors:FG Color")) -> ()  [unwired: 2 in, 2 out]
                n423 = To Long Integer(number=w735) -> (32bit integer=w734:i32)
                n424 = call "HT3_Finish.vi"("FileHeaderPos"=w731, "Rates"=w723, "Stop Reason"=w733, "error in"=w738, "Num Records"=w736, "Stop After (ms)"=w734, "refnum in"=w737) -> ("error out"=w730:errorcluster)  [unwired: 4 in]
              }
            }
            n425 = local read "X-Position"() -> (w593:dbl)
            n426 = local read "Y-Position"() -> (w592:dbl)
            n427 = local read "Z-Position"() -> (w591:dbl)
            n428 = Subtract(x=w594, y=w593) -> (x-y=w590:dbl)
            n429 = Subtract(x=w594, y=w592) -> (x-y=w589:dbl)
            n430 = Subtract(x=w594, y=w591) -> (x-y=w588:dbl)
            n431 = global read "GlobalConAxisPI.vi" "Conn. Axes"() -> (w599:string[])
            n432 = call "AOTF-Trigger_1.vi"("Channel"="Laser  Profile", "error in (no error)"=w632, "Triggered"=bool ?, "lp"=w626, "ap"=w627) -> ("error out"=w633:errorcluster)  [unwired: 2 in]
            n433 = Build Array(w590, w589, w588) -> (w598:dbl[])
            n434 = call "MOV.vi"("System no."=w600, "Axes to move"=w599, "Position values"=w598, "error in"=w602) -> ("error out"=w601:errorcluster)  [unwired: 15 in]
          }
          frame #2 {
            w875 = i32 ?
            w880 = i32 ?
            w908 = i32 ?
            w936 = i32 ? ("dimension size")
            n435 = Index Array(array=w907) -> (element=w974:T34)  [unwired: 1 in]
            n436 = Unbundle By Name(w974) -> ("Dev"=w893:i32)
            n437 = Equal?(x=w949, y=T10 ? ("Task")) -> (x = y?=w845:bool)
            n438 = local read "concatenated string"() -> (w900:string)
            n439 = And(x=w845, y="Autopoint-Autofocus Z") -> (x .and. y?=w937:bool)
            n440 = Or(x="Point Defocussed Cam", y="Auto Defocussed Cam") -> (x .or. y?=w862:bool)
            n441 = Select(t="Auto Measurement Time (ms)", s=w845, f="Measurement Time") -> (s? t:f=w846:i32)
            n442 = local read "X-Position"() -> (w955:dbl)
            n443 = local read "Y-Position"() -> (w954:dbl)
            n444 = local read "Z-Position"() -> (w890:dbl)
            n445 = Select(t=string ? ("Measurement Type"), s=w845, f=string ? ("Measurement Type")) -> (s? t:f=w899:string)
            n446 = case shown="True" w862 {
              tunnel: [w976 w981] -> w855
              tunnel: w856 -> [w976 w982]
              tunnel: w846 -> [_ w979]
              frame #0 {
              }
              frame #1 {
                n447 = global read "GlobalSetGetConfigureCamera.vi" "Exposure"() -> (w977:sgl)
                n448 = Greater?(x=w977, y=w979) -> (0:w980:bool)
                n449 = case shown="False" w980 {
                  tunnel: w979 -> [_ w984]
                  tunnel: [w983 w984] -> w978
                  tunnel: w977 -> [w983 _]
                  frame #0 {
                  }
                  frame #1 {
                  }
                }
                n450 = call "PrepCamera.vi"("mesTime"=w978, "error out 2"=w982) -> ("error out"=w981:errorcluster)  [unwired: 25 in]
              }
            }
            n451 = Select(t=T10 ? ("Task"), s=w845, f=T25 ? ("Do Measurement")) -> (s? t:f=w948:T10)
            n452 = local read "NxtAutMesPoint"() -> (w894:i32)
            n453 = Multiply(x=w846, y=i32 ?) -> (x*y=w847:i32)
            n454 = local read "Pattern"() -> (w895:dbl[][])
            n455 = Concatenate Strings(w900, w899) -> (w898:string)
            n456 = Bundle("X-Position"=w955, "Y-Position"=w954, "Z-Position"=w890) -> (w939:T38)  [unwired: 1 in]
            n457 = call "MTS_AutoPointCords.vi"("Is Auto Point"=w845, "Cords In"=w939, "Next Auto Measure Point"=w894, "Pattern"=w895) -> ("Cords"=w926:T38)  [unwired: 7 in]
            n458 = Unbundle By Name(w926) -> ("X-Position"=w866:dbl, "Y-Position"=w867:dbl, "Z-Position"=w876:dbl)
            n459 = Subtract(x=w880, y=w867) -> (x-y=w879:dbl)
            n460 = Subtract(x=w880, y=w866) -> (x-y=w878:dbl)
            n461 = Subtract(x=w880, y=w876) -> (x-y=w877:dbl)
            n462 = local read "PI SystemNumber"() -> (w888:i32)
            n463 = global read "GlobalConAxisPI.vi" "Conn. Axes"() -> (w882:string[])
            n464 = Build Array(w879, w878, w877) -> (w881:dbl[])
            n465 = local read "Last Image File No"() -> (w942:i32)
            n466 = call "MOV.vi"("System no."=w888, "Axes to move"=w882, "Position values"=w881, "No.of digits"=i16 ?, "error in"=w857) -> ("error out"=w870:errorcluster)  [unwired: 14 in]
            n467 = flat-sequence {
              tunnel: w870 -> [w985]
              tunnel: [w985] -> w869
              frame #0 {
                n468 = Wait (ms)(milliseconds to wait=u32 ?) -> ()  [unwired: 1 out]
              }
            }
            n469 = Select(t=T29 ? ("Measurement Type"), s=w845, f=T29 ? ("Measurement Type")) -> (s? t:f=w943:T29)
            n470 = Select(t=w942, s=w845, f=i32 ?) -> (s? t:f=w940:i32)
            n471 = local read "Workspace"() -> (w964:path)
            n472 = call "MTS_GenFileComment.vi"("Measurement Type"=w943, "Parent File No"=w940, "Info"=w904, "Upper Left"=w926, "error in"=w855) -> ("Comment"=w965:string, "error out"=w963:errorcluster)  [unwired: 7 in, 2 out]
            n473 = Not(x="Adjustment") -> (.not. x?=w902:bool)
            n474 = call "MTS_GetNextFileName.vi"("error in (no error)"=w963, "File Type"=string ?, "Measurement Type"=w898, "Workspace"=w964) -> ("error out"=w958:errorcluster, "Next File Name"=w957:path)  [unwired: 6 in]
            n475 = local read "CFD Settings"() -> (w933:T7)
            n476 = case shown="True" w902 {
              tunnel: w958 -> [w999 w1007]
              tunnel: w957 -> [_ w1006]
              tunnel: [w999 w1005] -> w858
              tunnel: [path ? w1000] -> w956
              tunnel: w943 -> [_ w1002]
              tunnel: w940 -> [_ w1004]
              tunnel: w938 -> [_ w1001]
              frame #0 {
              }
              frame #1 {
                n477 = call "MTS_AddFileToWorkspace.vi"("File Name"=w1006, "File Type"=T30 ?, "Measurement Type"=w1002, "error in (no error)"=w1007, "Parent"=w1004, "Tree Refnum"=w1001) -> ("File Name (dup)"=w1000:path, "error out"=w1005:errorcluster)  [unwired: 7 in, 1 out]
              }
            }
            n478 = call "POS?.vi"("System no."=w888, "Axes to query"=w882, "All axes?"=bool ?, "error in"=w869) -> ("Position"=w886:dbl[], "error out"=w889:errorcluster)  [unwired: 14 in]
            n479 = call "HH_Set.vi"("Device List"=w907, "CFD Settings"=w933, "error in (no error)"=w889) -> ("ht3 header out"=w953:T35, "Sync Rate"=w923:i32, "error out"=w951:errorcluster)  [unwired: 8 in, 2 out]
            n480 = Index Array(array=w886, index #1=i32 ? ("index"), index #2=i32 ? ("index"), index #3=i32 ? ("index")) -> (element #1=w874:dbl, element #2=w873:dbl, element #3=w872:dbl)
            n481 = Bundle By Name(cluster=w953, "AcquisitionTime (ms)"=w847) -> (w952:T35)
            n482 = Divide(x=i32 ? ("n"), y=w923) -> (x/y=w924:dbl)
            n483 = Subtract(x=w875, y=w874) -> (x-y=w844:dbl)
            n484 = Subtract(x=w875, y=w872) -> (x-y=w871:dbl)
            n485 = Subtract(x=w875, y=w873) -> (x-y=w843:dbl)
            n486 = property on="y-position" class="DigNum (strict)"("Value"=w844) -> ()  [unwired: 2 in, 2 out]
            n487 = property on="z-position" class="DigNum (strict)"("Value"=w871) -> ()  [unwired: 2 in, 2 out]
            n488 = case shown="True" w937 {
              tunnel: w951 -> [w1008 w1016]
              tunnel: [w1008 w1015] -> w950
              tunnel: w888 -> [_ w1010]
              tunnel: w924 -> [_ w1014]
              tunnel: w926 -> [_ w1013]
              tunnel: w893 -> [_ w1009]
              frame #0 {
              }
              frame #1 {
                # "Auto Z"
                n489 = call "MTS_AutoZPos.vi"("PH Dev"=w1009, "OFlow Interv [s]"=w1014, "PI System no."=w1010, "error in"=w1016, "Start Point"=w1013) -> ("New Z"=w1012:dbl, "Counts"=→"Counts":u32[], "error out"=w1015:errorcluster)  [unwired: 7 in, 1 out]
                n490 = local write "Z-Position"(w1012) -> ()
              }
            }
            n491 = property on="x-position" class="DigNum (strict)"("Value"=w843) -> ()  [unwired: 2 in, 2 out]
            n492 = Initialize Array(u32 ?, w936) -> (w968:u32[])
            n493 = global read "ccdChipPixels.vi" "CCD Chip horizontal start"() -> (w853:i32)
            n494 = global read "ccdChipPixels.vi" "CCD Chip horizontal end"() -> (w854:i32)
            n495 = global read "ccdChipPixels.vi" "CCD Chip Vertical Start"() -> (w851:i32)
            n496 = global read "ccdChipPixels.vi" "CCD Chip Vertical end"() -> (w852:i32)
            n497 = Subtract(x=w854, y=w853) -> (x-y=w849:i32)
            n498 = Subtract(x=w852, y=w851) -> (x-y=w848:i32)
            n499 = flat-sequence {
              tunnel: w971 -> [w1021]
              tunnel: w859 -> [w1038]
              tunnel: [w1019] -> w970
              tunnel: [w1035] -> w906
              tunnel: w967 -> [w1040]
              tunnel: w966 -> [w1031]
              tunnel: w960 -> [w1034]
              tunnel: w959 -> [w1033]
              tunnel: w935 -> [w1030]
              tunnel: w928 -> [w1027]
              tunnel: w927 -> [w1026]
              tunnel: w862 -> [w1018]
              frame #0 {
                # "Finish after Measurement"
                n500 = case shown="False" w1018 {
                  tunnel: w1021 -> [w1042 w1047]
                  tunnel: [w1042 w1044] -> w1020
                  frame #0 {
                  }
                  frame #1 {
                    n501 = call "SetShutter.vi"("type"=T17 ?, "mode"=T18 ?, "error in (no error)"=w1047) -> ("error out"=w1049:errorcluster)  [unwired: 11 in, 1 out]
                    n502 = call <vilib>:"Clear Errors.vi"("error in (no error)"=w1049) -> ("error out"=w1048:errorcluster)  [unwired: 6 in]
                    n503 = call "AbortAcquisition.vi"("error in (no error)"=w1048) -> ("error out"=w1043:errorcluster)  [unwired: 1 in, 1 out]
                    n504 = call <vilib>:"Clear Errors.vi"("error in (no error)"=w1043) -> ("error out"=w1044:errorcluster)  [unwired: 6 in]
                  }
                }
                n505 = Or(x=w1031, y=w1040) -> (x .or. y?=w1039:bool)
                n506 = Index Array(array=w1027, index=i32 ?) -> (element=w1028:dbl)
                n507 = case shown="False" w1039 {
                  tunnel: w1038 -> [w1051 w1052]
                  tunnel: [w1051 w1052] -> w1036
                  tunnel: [enum16{"timeover", "manual", "overflow"} ? ("Stop Reason") w1055] -> w1032
                  tunnel: w1031 -> [_ w1053]
                  frame #0 {
                  }
                  frame #1 {
                    n508 = Select(t=enum16{"timeover", "manual", "overflow"} ? ("Stop Reason"), s=w1053, f=enum16{"timeover", "manual", "overflow"} ? ("Stop Reason")) -> (s? t:f=w1055:enum16{"timeover", "manual", "overflow"})
                  }
                }
                n509 = Divide(x=w1026, y=w1028) -> (x/y=w1025:dbl)
                n510 = Multiply(x=i32 ?, y=w1025) -> (x*y=w1023:dbl)
                n511 = To Long Integer(number=w1023) -> (32bit integer=w1022:i32)
                n512 = property on="Point Measurement" class="Bool"("BoolText.Text"=string ? ("Caption.Text"), "BoolText.TextColor"=u32 ? ("Boolean Text.Colors:FG Color")) -> ()  [unwired: 2 in, 2 out]
                n513 = call "HT3_Finish.vi"("FileHeaderPos"=w1030, "Rates"=w1027, "Stop Reason"=w1032, "error in"=w1036, "Num Records"=w1033, "Stop After (ms)"=w1022, "refnum in"=w1034) -> ("error out"=w1035:errorcluster)  [unwired: 4 in]
                n514 = Build Array(w1021, w1020) -> (w1017:errorcluster[])
                n515 = call <vilib>:"Merge Errors.vi"("error array in"=w1017) -> ("error out"=w1019:errorcluster)  [unwired: 6 in]
              }
            }
            n516 = local read "Laser  Profile"() -> (w922:string)
            n517 = String To Byte Array(string=w922) -> (unsigned byte array=w920:u8[])
            n518 = Subtract(x=w920, y=i32 ?) -> (x-y=w915:i32[])
            n519 = String Length(string=w922) -> (length=w912:i32)
            n520 = Initialize Array(i32 ?, i32 ?, i32 ?) -> (w916:i32[][])
            n521 = Replace Array Subset(array=w916, new element=w915, index (col)=w908) -> (w914:i32[][])  [unwired: 1 in]
            n522 = Array Subset(array=w913, index=w908, length=w912) -> (w911:i32[])
            n523 = Replace Array Subset(array=w914, new element=w911, index (col)=i32 ?) -> (w910:i32[][])  [unwired: 1 in]
            n524 = call "HT3_Create.vi"("Laser"=w910, "Save pt3"=w902, "error in"=w950, "Comment"=w965, "ht3 Header in"=w952, "File Path"=w956) -> ("error out"=w891:errorcluster, "FileHeaderPos"=w935:T37, "refnum out"=w961:refnum<file>)  [unwired: 3 in]
            n525 = call "HH_Start.vi"("Device Index"=w893, "Acq. Time"=w847, "error in (no error)"=w891) -> ("error out"=w861:errorcluster)  [unwired: 11 in, 1 out]
            n526 = case shown="True" w862 {
              tunnel: [w987 w991] -> w841
              tunnel: w891 -> [w987 w990]
              tunnel: w845 -> [_ w989]
              tunnel: [_ w988] -> w850
              frame #0 {
              }
              frame #1 {
                n527 = control-ref of="NxtAutMesPoint"() -> (w996:refnum<vi>)
                n528 = control-ref of="Workspace"() -> (w997:refnum<vi>)
                n529 = control-ref of="y-position"() -> (w993:refnum<vi>)
                n530 = control-ref of="x-position"() -> (w994:refnum<vi>)
                n531 = control-ref of="z-position"() -> (w992:refnum<vi>)
                n532 = control-ref of="Pattern"() -> (w995:refnum<vi>)
                n533 = call "DefocussedImage.vi"("Path in"=w997, "reference"=w996, "Boolean"=w989, "reference 2"=w995, "reference 3"=w994, "error in (no error)"=w990, "reference 4"=w993, "reference 5"=w992) -> ("camout"=w988:i32[], "error out"=w991:errorcluster)  [unwired: 6 in]
              }
            }
            n534 = Unbundle By Name(w861) -> ("status"=w973:bool)
            n535 = Not(x=w973) -> (.not. x?=w972:bool)
            n536 = case shown="True" w972 {
              tunnel: [w1063 w1066] -> w860
              tunnel: w861 -> [w1064 w1075]
              tunnel: w858 -> [w1065 w1086]
              tunnel: [w1065 w1085] -> w971
              tunnel: w893 -> [w1058 w1074]
              tunnel: w968 -> [_ w1082]
              tunnel: w936 -> [_ w1081]
              tunnel: [w1062 w1080] -> w967
              tunnel: [w1062 w1079] -> w966
              tunnel: w961 -> [w1061 w1078]
              tunnel: [w1061 w1077] -> w960
              tunnel: [i64 ? ("Num Records Total") w1076] -> w959
              tunnel: [dbl[] ? w1071] -> w928
              tunnel: [i32 ? w1070] -> w927
              frame #0 {
                w1062 = bool ? ("Stop Measurement")
                n537 = call "HH_Stop.vi"("Device Index"=w1058, "error in (no error)"=w1064) -> ("error out"=w1063:errorcluster)  [unwired: 12 in, 1 out]
              }
              frame #1 {
                # "Overflow Interv. Time (s)"
                # "No Error"
                n538 = Initialize Array(i32 ?, i32 ?) -> (w1069:i32[])
                n539 = while {
                  tunnel: w1074 -> [w1095]
                  tunnel: w1082 -> [w1119]
                  tunnel: w1081 -> [w1118]
                  shift-right: [w1096] -> w1084
                  shift-left: w1075 -> [w1120]
                  shift-right: [w1117] -> w1085
                  shift-left: w1086 -> [w1117]
                  shift-right: [bool ? ("Reset")] -> _
                  shift-left: bool ? ("Reset") -> [w1113]
                  tunnel: [w1110] -> w1080
                  tunnel: [w1102] -> w1079
                  tunnel: w1078 -> [w1106]
                  tunnel: [w1105] -> w1077
                  tunnel: [w1104] -> w1076
                  tunnel: [w1103] -> w1070
                  shift-right: [w1090] -> w1072
                  shift-left: w1069 -> [w1089]
                  tunnel: [w1087] -> w1073
                  i -> [w1088]
                  stop <- w1116 stop-if-true
                  n540 = call "HH_FIFORead.vi"("Device Index"=w1095, "Buffer In"=w1119, "Count"=w1118, "error in (no error)"=w1120) -> ("OK"=w1111:bool, "Buffer Out"=w1107:u32[], "Data Count"=w1108:i32, "FiFo Overrun"=w1110:bool, "error out"=w1109:errorcluster)  [unwired: 7 in]
                  n541 = Wait (ms)(milliseconds to wait=u32 ?) -> ()  [unwired: 1 out]
                  n542 = Unbundle(w1109) -> ("status"=w1115:bool)  [unwired: 2 out]
                  n543 = local write "Buffer Overrun"(w1110) -> ()
                  n544 = call "HT3_Write.vi"("error in"=w1109, "Data Count"=w1108, "Data in"=w1107, "refnum in"=w1106) -> ("error out"=w1097:errorcluster, "refnum out"=w1105:refnum<file>)  [unwired: 6 in]
                  n545 = call "HH_TraceAndHisto.vi"("Data In"=w1107, "Reset"=w1113, "Data Count"=w1108) -> ("Histograms"=w1099:i32[][], "Total Oveflow Count"=w1103:u64, "Num Records Total"=w1104:i64, "Traces"=w1098:i32[][])  [unwired: 8 in, 1 out]
                  n546 = local read "Stop Measurement"() -> (w1101:bool)
                  n547 = local read "Global Stop"() -> (w1100:bool)
                  n548 = local write "Trace"(w1098) -> ()
                  n549 = call "GetCountRates.vi"("error in (no error)"=w1097, "DeviceIndex"=w1095) -> ("error out"=w1096:errorcluster, "CntRates"=w1091:dbl[], "SyncRate"=w1092:i32)  [unwired: 1 in]
                  n550 = Compound Arithmetic op=OR(invert w1111, w1115, w1100, w1101) -> (w1116:bool)
                  n551 = local write "Histogram"(w1099) -> ()
                  n552 = Insert Into Array(array=w1091, index=i32 ?, new element=w1092) -> (w1093:dbl[])
                  n553 = Or(x=w1101, y=w1100) -> (x .or. y?=w1102:bool)
                  n554 = Add(x=w1089, y=w1093) -> (x+y=w1090:dbl[])
                  n555 = Increment(x=w1088) -> (x+1=w1087:i32)
                }
                n556 = Divide(x=w1072, y=w1073) -> (x/y=w1071:dbl[])
                n557 = call "HH_Stop.vi"("Device Index"=w1074, "error in (no error)"=w1084) -> ("error out"=w1066:errorcluster)  [unwired: 12 in, 1 out]
              }
            }
            n558 = Reshape Array(w850, w849, w848) -> (w842:i32[][])
            n559 = property on="Point" class="IntGraph (strict)"(error in=w841, "Value"=w842) -> (error out=w840:errorcluster)  [unwired: 1 in, 1 out]
            n560 = Build Array(w860, w840) -> (w839:errorcluster[])
            n561 = call <vilib>:"Merge Errors.vi"("error array in"=w839) -> ("error out"=w859:errorcluster)  [unwired: 6 in]
            n562 = call "AOTF-Trigger_1.vi"("Channel"=w922, "Pulse length"=w913, "Sync trigger ratio"=i32 ?, "error in (no error)"=w857, "Triggered"=bool ?) -> ("error out"=w931:errorcluster)  [unwired: 2 in]
            n563 = call "MOV.vi"("System no."=w888, "Axes to move"=w882, "Position values"=w881, "error in"=w906) -> ("error out"=w905:errorcluster)  [unwired: 15 in]
          }
          frame #3 {
            n564 = local read "Active pt3"() -> (w1128:path)
            n565 = call "MTS_GetFileFromWS.vi"(".pt3 File Name"=w1128) -> ("File Header"=w1127:T39)  [unwired: 9 in, 1 out]
            n566 = Unbundle By Name(w1127) -> ("Measurement Type"=w1126:T40, "Pixels"=w1123:i32[])
            n567 = control-ref of="WS File Tree"() -> (w1129:refnum<vi>)
            n568 = Equal?(x=T29 ? ("Measurement Type"), y=w1126) -> (x = y?=w1124:bool)
            n569 = case shown="True" w1124 {
              tunnel: w1132 -> [w1133 w1156]
              tunnel: w1128 -> [_ w1155]
              tunnel: w1128 -> [_ _]
              tunnel: [w1133 w1135] -> w1121
              tunnel: w1129 -> [_ _]
              tunnel: w1123 -> [_ w1140]
              frame #0 {
              }
              frame #1 {
                # "Image Intensity Array"
                # "Image Intensity Array"
                n570 = call "HT3_Open.vi"("error in"=w1156, "File Path"=w1155) -> ("error out"=w1148:errorcluster, "Header"=w1152:T41, "refnum out"=w1154:refnum<file>)  [unwired: 3 in, 4 out]
                n571 = Unbundle By Name(w1152) -> ()  [unwired: 15 out]
                n572 = Index Array(array=w1140, index #2=i32 ? ("index")) -> (element #1=w1137:i32, element #2=w1138:i32)  [unwired: 1 in]
                n573 = Initialize Array(i32 ? ("element"), w1137, w1138) -> (w1150:i32[][])
                n574 = Initialize Array(i32 ? ("element"), i32 ? ("dimension size"), w1137, w1138) -> (w1143:i32[][][])
                n575 = while {
                  tunnel: w1154 -> [w1181]
                  shift-right: [bool ? ("Start From Top")] -> _
                  shift-left: bool ? ("Start From Top") -> [w1175]
                  shift-right: [w1174] -> w1147
                  shift-left: w1148 -> [w1172]
                  tunnel: [w1173] -> w1146
                  tunnel: w1150 -> [w1171]
                  tunnel: [w1170] -> w1149
                  tunnel: [w1171] -> _
                  stop <- w1178 stop-if-true
                  n576 = call "HT3_Read.vi"("Start From Top"=w1175, "error in"=w1172, "Data count"=i32 ?, "refnum in"=w1181) -> ("error out"=w1174:errorcluster, "Data out"=w1177:u32[], "refnum out"=w1173:refnum<file>, "EOF?"=w1178:bool)  [unwired: 4 in]
                  n577 = Array Size(array=w1177) -> (size(s)=w1176:i32)
                  n578 = call "HH_FileToImage_1.vi"("Data In"=w1177, "Reset"=w1175, "Data Count"=w1176) -> ("Histograms"=w1170:i32[][])  [unwired: 7 in, 5 out]
                }
                n579 = call "MTS_SelectTCSPCBinning.vi"("Histograms in"=w1149) -> ("TCSPC Binning"=w1142:i32[][])  [unwired: 1 in, 9 out]
                n580 = while {
                  tunnel: w1146 -> [w1169]
                  shift-right: [bool ? ("Start From Top")] -> _
                  shift-left: bool ? ("Start From Top") -> [w1163]
                  shift-right: [w1162] -> w1134
                  shift-left: w1147 -> [w1158]
                  tunnel: [w1161] -> w1136
                  tunnel: w1143 -> [w1160]
                  tunnel: [w1159] -> _
                  tunnel: w1142 -> [w1157]
                  stop <- w1166 stop-if-true
                  n581 = call "HT3_Read.vi"("Start From Top"=w1163, "error in"=w1158, "Data count"=i32 ?, "refnum in"=w1169) -> ("error out"=w1162:errorcluster, "Data out"=w1165:u32[], "refnum out"=w1161:refnum<file>, "EOF?"=w1166:bool)  [unwired: 4 out]
                  n582 = Array Size(array=w1165) -> (size(s)=w1164:i32)
                  n583 = call "HH_ToColorImage.vi"("Data In"=w1165, "Reset"=w1163, "Image Array In"=w1160, "Data Count"=w1164, "TCSPC Binning"=w1157) -> ("Image Array Out"=w1159:i32[][][])  [unwired: 2 in, 8 out]
                }
                n584 = Close File(refnum=w1136, error in=w1134) -> (error out=w1135:errorcluster)  [unwired: 1 out]
              }
            }
          }
          frame #4 {
            # "dirty trick"
            n585 = local read "Active pt3"() -> (w1208:path)
            n586 = call "MTS_GetFileFromWS.vi"(".pt3 File Name"=w1208) -> ("File Header"=w1207:T39)  [unwired: 9 in, 1 out]
            n587 = Unbundle By Name(w1207) -> ("Measurement Type"=w1206:T40, "Pixels"=w1194:i32[], "Upper Left"=w1203:T42, "Scan Axis"=w1202:enum32{"x-y", "x-z", "y-z"})
            n588 = local read "Picture size 2"() -> (w1189:dbl)
            n589 = local read "Picture size"() -> (w1192:dbl)
            n590 = local read "Resolution"() -> (w1190:dbl)
            n591 = local read "X-Position"() -> (w1183:dbl)
            n592 = local read "Y-Position"() -> (w1182:dbl)
            n593 = Divide(x=w1192, y=w1190) -> (x/y=w1191:dbl)
            n594 = Divide(x=w1189, y=w1190) -> (x/y=w1188:dbl)
            n595 = Equal?(x=T29 ? ("Measurement Type"), y=w1206) -> (x = y?=w1204:bool)
            n596 = call "MTS_ScannerXYZToImageXY.vi"("Axis"=w1202, "Scanner XYZ"=w1203) -> ("Image Y"=w1185:dbl, "Image X"=w1187:dbl)
            n597 = case shown="True" bool ? {
              tunnel: [w1211 w1214] -> w1193
              tunnel: w1194 -> [w1211 _]
              tunnel: w1191 -> [_ w1218]
              tunnel: w1188 -> [_ w1217]
              tunnel: [w1210 w1213] -> w1186
              tunnel: w1187 -> [w1210 _]
              tunnel: [w1209 w1212] -> w1184
              tunnel: w1185 -> [w1209 _]
              tunnel: w1183 -> [_ w1213]
              tunnel: w1182 -> [_ w1212]
              frame #0 {
              }
              frame #1 {
                n598 = To Long Integer(number=w1218) -> (32bit integer=w1216:i32)
                n599 = To Long Integer(number=w1217) -> (32bit integer=w1215:i32)
                n600 = Build Array(w1216, w1215) -> (w1214:i32[])
              }
            }
            n601 = Build Array(w1192, w1189) -> (w1198:dbl[])
            n602 = case shown="True" w1204 {
              tunnel: w1201 -> [w1219 w1295]
              tunnel: w1208 -> [_ _]
              tunnel: w1208 -> [_ _]
              tunnel: [w1219 w1300] -> w1199
              tunnel: w1193 -> [_ w1317]
              tunnel: w1198 -> [_ w1299]
              tunnel: w1186 -> [_ w1309]
              tunnel: w1184 -> [_ w1310]
              frame #0 {
              }
              frame #1 {
                w1269 = T11 ? items=["Center of Mass X", "Center of Mass Y", "First Pixel X", "First Pixel Y", "Bounding Rect Left", "Bounding Rect Top", "Bounding Rect Right", "Bounding Rect Bottom", "Max Feret Diameter Start X", "Max Feret Diameter Start Y", "Max Feret Diameter End X", "Max Feret Diameter End Y", "Max Horiz. Segment Length Left", "Max Horiz. Segment Length Right", "Max Horiz. Segment Length Row", "-", "Bounding Rect Width", "Bounding Rect Height", "Bounding Rect Diagonal", "Perimeter", "Convex Hull Perimeter", "Holes' Perimeter", "Max Feret Diameter", "Equivalent Ellipse Major Axis", "Equivalent Ellipse Minor Axis", "Equivalent Ellipse Minor Axis (Feret)", "Equivalent Rect Long Side", "Equivalent Rect Short Side", "Equivalent Rect Diagonal", "Equivalent Rect Short Side (Feret)", "Average Horiz. Segment Length", "Average Vert. Segment Length", "Hydraulic Radius", "Waddel Disk Diameter", "-", "Area", "Holes' Area", "Particle & Holes' Area", "Convex Hull Area", "Image Area", "-", "Number of Holes", "Number of Horiz. Segments", "Number of Vert. Segments", "-", "Orientation", "Max Feret Diameter Orientation", "-", "% Area/Image Area", "% Area/(Particle & Holes' Area)", "Ratio of Equivalent Ellipse Axes", "Ratio of Equivalent Rect Sides", "-", "Elongation Factor", "Compactness Factor", "Heywood Circularity Factor", "Type Factor", "-", "Sum X", "Sum Y", "Sum XX", "Sum XY", "Sum YY", "Sum XXX", "Sum XXY", "Sum XYY", "Sum YYY", "-", "Moment of Inertia XX", "Moment of Inertia XY", "Moment of Inertia YY", "Moment of Inertia XXX", "Moment of Inertia XXY", "Moment of Inertia XYY", "Moment of Inertia YYY", "Norm. Moment of Inertia XX", "Norm. Moment of Inertia XY", "Norm. Moment of Inertia YY", "Norm. Moment of Inertia XXX", "Norm. Moment of Inertia XXY", "Norm. Moment of Inertia XYY", "Norm. Moment of Inertia YYY", "Hu Moment 1", "Hu Moment 2", "Hu Moment 3", "Hu Moment 4", "Hu Moment 5", "Hu Moment 6", "Hu Moment 7"] ("Measurement Parameter")
                w1250 = bool ? ("Measurement Type")
                w1274 = T11 ? items=["Center of Mass X", "Center of Mass Y", "First Pixel X", "First Pixel Y", "Bounding Rect Left", "Bounding Rect Top", "Bounding Rect Right", "Bounding Rect Bottom", "Max Feret Diameter Start X", "Max Feret Diameter Start Y", "Max Feret Diameter End X", "Max Feret Diameter End Y", "Max Horiz. Segment Length Left", "Max Horiz. Segment Length Right", "Max Horiz. Segment Length Row", "-", "Bounding Rect Width", "Bounding Rect Height", "Bounding Rect Diagonal", "Perimeter", "Convex Hull Perimeter", "Holes' Perimeter", "Max Feret Diameter", "Equivalent Ellipse Major Axis", "Equivalent Ellipse Minor Axis", "Equivalent Ellipse Minor Axis (Feret)", "Equivalent Rect Long Side", "Equivalent Rect Short Side", "Equivalent Rect Diagonal", "Equivalent Rect Short Side (Feret)", "Average Horiz. Segment Length", "Average Vert. Segment Length", "Hydraulic Radius", "Waddel Disk Diameter", "-", "Area", "Holes' Area", "Particle & Holes' Area", "Convex Hull Area", "Image Area", "-", "Number of Holes", "Number of Horiz. Segments", "Number of Vert. Segments", "-", "Orientation", "Max Feret Diameter Orientation", "-", "% Area/Image Area", "% Area/(Particle & Holes' Area)", "Ratio of Equivalent Ellipse Axes", "Ratio of Equivalent Rect Sides", "-", "Elongation Factor", "Compactness Factor", "Heywood Circularity Factor", "Type Factor", "-", "Sum X", "Sum Y", "Sum XX", "Sum XY", "Sum YY", "Sum XXX", "Sum XXY", "Sum XYY", "Sum YYY", "-", "Moment of Inertia XX", "Moment of Inertia XY", "Moment of Inertia YY", "Moment of Inertia XXX", "Moment of Inertia XXY", "Moment of Inertia XYY", "Moment of Inertia YYY", "Norm. Moment of Inertia XX", "Norm. Moment of Inertia XY", "Norm. Moment of Inertia YY", "Norm. Moment of Inertia XXX", "Norm. Moment of Inertia XXY", "Norm. Moment of Inertia XYY", "Norm. Moment of Inertia YYY", "Hu Moment 1", "Hu Moment 2", "Hu Moment 3", "Hu Moment 4", "Hu Moment 5", "Hu Moment 6", "Hu Moment 7"] ("Measurement Parameter")
                w1289 = T43 ? items=["Grayscale (U8)", "Grayscale (I16)", "Grayscale (SGL)", "Complex (CSG)", "RGB (U32)", "HSL (U32)", "RGB (U64)", "Grayscale (U16)"] ("Image Type")
                w1297 = T43 ? items=["Grayscale (U8)", "Grayscale (I16)", "Grayscale (SGL)", "Complex (CSG)", "RGB (U32)", "HSL (U32)", "RGB (U64)", "Grayscale (U16)"] ("Image Type")
                w1316 = i32 ? ("index")
                # "Pixel Size [um]"
                n603 = Index Array(array=w1299, index #2=w1316) -> (element #1=w1315:dbl, element #2=w1312:dbl)  [unwired: 1 in]
                n604 = Index Array(array=w1317, index #2=w1316) -> (element #1=w1314:i32, element #2=w1313:i32)  [unwired: 1 in]
                n605 = Divide(x=w1315, y=w1314) -> (x/y=w1221:dbl)
                n606 = Divide(x=w1312, y=w1313) -> (x/y=w1311:dbl)
                n607 = Reciprocal(x=w1221) -> (1/x=w1226:dbl)
                n608 = Multiply(x=w1226, y="Focuswidth") -> (x*y=w1225:dbl)
                n609 = Random Number (0-1)() -> (number: 0 to 1=w1294:dbl)
                n610 = Number To Decimal String(number=w1294) -> (decimal integer string=w1293:string)  [unwired: 1 in]
                n611 = Concatenate Strings(w1293, string ? ("Image Name")) -> (w1291:string)
                n612 = call "IMAQ Create"("Image Name"=w1291, "Image Type"=w1297, "error in (no error)"=w1295) -> ("New Image"=w1296:T5, "error out"=w1284:errorcluster)  [unwired: 2 in]
                n613 = local read "Image"() -> (w1228:i32[][])
                n614 = call "MTS_IntensityArrayToImage.vi"(0:"Image"=w1296, 1:"Image"=w1228, "error in (no error)"=w1284, "Log Scale"=bool ?) -> ("Image Out"=w1249:T5, "error out"=w1241:errorcluster)  [unwired: 10 in]
                n615 = Random Number (0-1)() -> (number: 0 to 1=w1288:dbl)
                n616 = Array To Cluster(array=T32 ? ("MesaurementSelection")) -> (cluster=w1277:T44)
                n617 = Number To Decimal String(number=w1288) -> (decimal integer string=w1287:string)  [unwired: 1 in]
                n618 = Unbundle By Name(w1277) -> ("MesaurementSelection[0]"=w1275:T45, "MesaurementSelection[1]"=w1270:T45, "MesaurementSelection[2]"=w1265:T45, "MesaurementSelection[3]"=w1256:T45)
                n619 = Concatenate Strings(w1287, string ? ("Image Name")) -> (w1285:string)
                n620 = call "IMAQ Create"("Image Name"=w1285, "Image Type"=w1289, "error in (no error)"=w1241) -> ("New Image"=w1283:T5, "error out"=w1240:errorcluster)  [unwired: 2 in]
                n621 = Bundle By Name(cluster=w1275, "Measurement Parameter"=w1274, "Range Lower Value"="X Start 2", "Range Upper Value"="X End 2", "Range"="Exclude / Include X", "Measurement Type"=w1250) -> (w1264:T45)
                n622 = Bundle By Name(cluster=w1270, "Measurement Parameter"=w1269, "Range Lower Value"="Y Start 2", "Range Upper Value"="Y End 2", "Range"="Exclude / Include Y", "Measurement Type"=w1250) -> (w1263:T45)
                n623 = Bundle By Name(cluster=w1265, "Measurement Parameter"="Measurement Parameter 1", "Range Lower Value"="Range Lower Value Par 1", "Range Upper Value"="Range Upper Value  Par 1", "Range"="Ex/In Par 1", "Measurement Type"=w1250) -> (w1262:T45)
                n624 = Bundle By Name(cluster=w1256, "Measurement Parameter"="Measurement Parameter 2", "Range Lower Value"="Range Lower Value Par 2", "Range Upper Value"="Range Upper Value Par 2", "Range"="Ex/In Par 2", "Measurement Type"=w1250) -> (w1255:T45)
                n625 = Build Array(w1264, w1263, w1262, w1255) -> (w1261:T32)
                n626 = call "MTS_IntensityArrayToImage.vi"(0:"Image"=w1283, 1:"Image"=w1228, "error in (no error)"=w1240, "Log Scale"=bool ?) -> ("Image Out"=w1234:T5, "error out"=w1239:errorcluster)  [unwired: 10 in]
                n627 = case shown="0, Default" "Detection Modus" {
                  tunnel: "Remove Outliers" -> [_ w1351]
                  tunnel: [w1328 w1342] -> w1290
                  tunnel: w1239 -> [w1333 w1350]
                  tunnel: [w1326 w1340] -> w1281
                  tunnel: "Filter" -> [_ w1349]
                  tunnel: w1261 -> [_ w1348]
                  tunnel: w1249 -> [_ w1343]
                  tunnel: path ? ("Template File Path (GeometricMatching)") -> [_ _]
                  tunnel: "Settings (GeometricMatching)" -> [_ _]
                  tunnel: T31 ? ("Rounding Mode Gaussian") -> [_ w1347]
                  tunnel: T31 ? ("Rounding Mode Convolution") -> [_ w1346]
                  tunnel: "Square/Hexa" -> [_ w1345]
                  tunnel: "Connectivity 4/8" -> [_ w1344]
                  tunnel: w1234 -> [w1330 w1338]
                  tunnel: [w1330 w1335] -> w1238
                  tunnel: [w1332 w1336] -> w1236
                  tunnel: "Manual" -> [_ w1334]
                  tunnel: w1228 -> [w1324 _]
                  tunnel: "Mode" -> [w1323 _]
                  tunnel: w1225 -> [w1322 _]
                  tunnel: [w1321 _] -> w1223
                  tunnel: "NA" -> [w1320 _]
                  tunnel: w1221 -> [w1319 _]
                  tunnel: "TSH" -> [w1318 _]
                  frame #0 {
                    n628 = To Double Precision Float(number=w1324) -> (double precision float=w1325:dbl[][])
                    n629 = script code="addpath(path);\nswitch (mode)\ncase 0\nmaskGauss = GenGauss2D(focus);\n[err,bim,cim,sim,yc,xc,bc,cc,sc,len,imm]=FindPatternCP(image,maskGauss,[],[],[],tsh);\npattern=maskGauss;\ncase 1\nmaskRad=Radialpattern_gen('radial', Pixel,NA);\n[err,bim,cim,sim,yc,xc,bc,cc,sc,len,imm]=FindPatternCP(image,maskRad,[],[],[],tsh);\npattern=maskRad(:,:,15);\ncase 2\nmaskAzi=Radialpattern_gen('azimuthal', Pixel,NA);\n[err,bim,cim,sim,yc,xc,bc,cc,sc,len,imm]=FindPatternCP(image,maskAzi,[],[],[],tsh);\npattern=maskAzi(:,:,15);\nend\nxc=xc-1;\nyc=yc-1;"("??"=w1333, "path"=string ?, "image"=w1325, "mode"=w1323, "focus"=w1322, "NA"=w1320, "Pixel"=w1319, "tsh"=w1318) -> ("??"=w1332:errorcluster, "pattern"=w1321:dbl[][], "xc"=w1329:dbl[], "yc"=w1327:dbl[])
                    n630 = Build Array(w1329, w1327) -> (w1328:dbl[][])
                    n631 = Array Size(array=w1327) -> (size(s)=w1326:i32)
                  }
                  frame #1 {
                    n632 = call "SingleMoleFinderEasy.vi"("Image Src"=w1343, "Number of Erosion"=w1351, "HolesBorder"=w1349, "Selection Values"=w1348, "Rounding Mode Gaussian"=w1347, "error in"=w1350, "Rounding Mode Convolution"=w1346, "Square/Hexa (Square)"=w1345, "Connectivity 4/8 (8)"=w1344) -> ("Number of Particles"=w1339:i32, "Particle Measurements (Pixels)"=w1341:dbl[][], "error out"=w1337:errorcluster)  [unwired: 15 in, 1 out]
                    n633 = case shown="True" w1334 {
                      tunnel: w1337 -> [w1355 w1363]
                      tunnel: [w1355 w1362] -> w1336
                      tunnel: [w1352 w1361] -> w1335
                      tunnel: [w1353 w1360] -> w1342
                      tunnel: w1341 -> [w1353 w1357]
                      tunnel: [w1354 w1359] -> w1340
                      tunnel: w1339 -> [w1354 w1358]
                      tunnel: w1338 -> [w1352 w1356]
                      frame #0 {
                      }
                      frame #1 {
                        n634 = while {
                          tunnel: w1363 -> [w1378]
                          tunnel: [w1377] -> w1362
                          tunnel: w1356 -> [w1376]
                          tunnel: [w1375] -> w1361
                          shift-right: [w1368] -> w1360
                          shift-left: w1357 -> [w1367]
                          tunnel: [w1366] -> w1359
                          tunnel: w1358 -> [w1365]
                          i -> [w1372]
                          stop <- w1374 stop-if-true
                          n635 = call "IMAQ Select Point"("Window Number (0...15)"=i32 ?, "error in (no error)"=w1378, "Image In"=w1376) -> ("error out"=w1377:errorcluster, "Cancelled"=w1374:bool, "Point"=w1373:T46, "Image Out (duplicate)"=w1375:T5)  [unwired: 5 in]
                          n636 = Unbundle(w1373) -> ("X"=w1371:sgl, "Y"=w1370:sgl)
                          n637 = Build Array(w1371, w1370) -> (w1369:sgl[])
                          n638 = Add(x=w1365, y=w1372) -> (x+y=w1366:i32)
                          n639 = Insert Into Array(array=w1367, index (row)=w1366, new element=w1369) -> (w1368:dbl[][])  [unwired: 1 in]
                        }
                      }
                    }
                  }
                }
                "Number of Particles" <- w1281
                "Image 2" <- w1223
                n640 = Index Array(array=w1290, index (col) #1=i32 ? ("index (row)"), index (col) #2=i32 ? ("index (col)")) -> (element #1=w1233:dbl[], element #2=w1231:dbl[])  [unwired: 2 in]
                n641 = Multiply(x=w1221, y=w1233) -> (x*y=w1308:dbl[])
                n642 = Multiply(x=w1231, y=w1311) -> (x*y=w1307:dbl[])
                n643 = To Word Integer(number=w1233) -> (16bit integer=w1232:i16[])
                n644 = To Word Integer(number=w1231) -> (16bit integer=w1230:i16[])
                n645 = Add(x=w1309, y=w1308) -> (x+y=w1303:dbl[])
                n646 = Add(x=w1307, y=w1310) -> (x+y=w1302:dbl[])
                n647 = for {
                  N: w1281 -> [_]
                  shift-right: [w1385] -> w1237
                  shift-left: w1238 -> [w1386]
                  tunnel: w1232 -> [w1384] mode=indexing
                  tunnel: w1230 -> [w1383] mode=indexing
                  shift-right: [w1387] -> w1235
                  shift-left: w1236 -> [w1388]
                  tunnel: u32 ? -> [w1382]
                  tunnel: dbl ? ("x") -> [w1381]
                  n648 = call "MTS_DrawCrossIMAQIamge.vi"("Image"=w1386, "Size"=w1381, "Color"=w1382, "X"=w1384, "Y"=w1383, "error in (no error)"=w1388) -> ("Image Out"=w1385:T5, "error out"=w1387:errorcluster)  [unwired: 8 in]
                }
                "AM image" <- w1237
                n649 = Build Array(w1303, w1302, w1232, w1230) -> (→"Pattern":dbl[][])
                n650 = flat-sequence {
                  tunnel: w1235 -> [w1380]
                  tunnel: [w1380] -> w1300
                  frame #0 {
                    n651 = local write "Tab Control"(T4 ? ("Tab Control")) -> ()
                  }
                }
                n652 = global write "patternImg.vi" "New Image"(w1237) -> ()
              }
            }
          }
          frame #5 {
            # "Init"
            n653 = local read "Pattern"() -> (w1399:dbl[][])
            n654 = Index Array(array=w1399, index (row) #1=i32 ? ("index (row)"), index (row) #2=i32 ? ("index (col)")) -> (element #1=w1396:dbl[], element #2=→"subarray":dbl[])  [unwired: 2 in]
            n655 = local read "NxtAutMesPoint"() -> (w1407:i32)
            n656 = Array Size(array=w1396) -> (size(s)=w1395:i32)
            n657 = Less Than 0?(x=w1407) -> (x < 0?=w1410:bool)
            n658 = case shown="False" w1410 {
              tunnel: w1404 -> [w1431 w1435]
              tunnel: [w1431 w1434] -> w1408
              tunnel: [w1430 w1432] -> w1406
              tunnel: w1395 -> [_ w1432]
              frame #0 {
                n659 = local read "Auto Measure Points"() -> (w1430:i32)
              }
              frame #1 {
                n660 = Number To Decimal String(number=w1432) -> (decimal integer string=w1437:string)  [unwired: 1 in]
                n661 = Concatenate Strings(string ? ("Caption.Text"), w1437) -> (w1436:string)
                n662 = property on="Auto Meas Progress" class="Slide (strict)"(error in=w1435, "Scale.Minimum"=dbl ? ("Scale.Range:Minimum"), "Scale.Maximum"=w1432, "Value"=i32 ? ("Auto Meas Progress"), "Caption.Text"=w1436) -> (error out=w1434:errorcluster)  [unwired: 1 in, 1 out]
                "Auto Measure Points" <- w1432
              }
            }
            n663 = Increment(x=w1407) -> (x+1=w1390:i32)
            "NxtAutMesPoint" <- w1390
            n664 = Greater Or Equal?(x=w1390, y=w1406) -> (x >= y?=w1409:bool)
            n665 = Increment(x=w1390) -> (x+1=w1405:i32)
            n666 = Index Array(array=w1399, index (row) #1=i32 ? ("index (row)"), index (col) #1=w1390, index (row) #2=i32 ? ("index (col)"), index (col) #2=w1390) -> (element #1=w1398:dbl, element #2=w1397:dbl)
            n667 = case shown="False" w1409 {
              tunnel: w1408 -> [w1421 w1429]
              tunnel: [w1427 w1429] -> w1402
              tunnel: [T14 ? ("Do Measurement") T14 ? ("Do Measurement")] -> w1401
              tunnel: w1405 -> [w1422 _]
              tunnel: w1398 -> [w1419 _]
              tunnel: w1397 -> [w1418 _]
              tunnel: w1406 -> [w1415 _]
              frame #0 {
                # "Prpare For Next Point"
                # "1 loc max  2 undef 0 saddle -1 local min"
                n668 = global read "patternImg.vi" "New Image"() -> (w1411:T5)
                n669 = Number To Decimal String(number=w1422) -> (decimal integer string=w1424:string)  [unwired: 1 in]
                n670 = Number To Decimal String(number=w1415) -> (decimal integer string=w1416:string)  [unwired: 1 in]
                n671 = Concatenate Strings(string ? ("Caption.Text"), w1424, string ? ("Caption.Text"), w1416) -> (w1423:string)
                n672 = call "MTS_DrawCrossIMAQIamge.vi"("Image"=w1411, "Size"=dbl ? ("x"), "Color"=u32 ?, "X"=w1419, "Y"=w1418, "error in (no error)"=w1421) -> ("Image Out"=w1412:T5, "error out"=w1420:errorcluster)  [unwired: 8 in]
                n673 = property on="Auto Meas Progress" class="Slide (strict)"(error in=w1420, "Value"=w1422, "Caption.Text"=w1423) -> (error out=w1427:errorcluster)  [unwired: 1 in, 1 out]
                n674 = local write "AM image"(w1412) -> ()
              }
              frame #1 {
                # "No More Points"
              }
            }
          }
        }
        n675 = local write "Buffer Overrun"(w574) -> ()
      }
      frame #1 {
      }
    }
    n676 = Unbundle(w559) -> ("status"=w558:bool)  [unwired: 2 out]
    n677 = flat-sequence {
      tunnel: w562 -> [w1455]
      tunnel: [w1455] -> w561
      tunnel: w557 -> [w1452]
      frame #0 {
        n678 = local write "Task"(w1452) -> ()
        n679 = Equal?(x=w1452, y=T25 ? ("Do Measurement")) -> (x = y?=w1453:bool)
        n680 = Not(x=w1453) -> (.not. x?=w1454:bool)
        n681 = local write "Running"(w1454) -> ()
      }
    }
    n682 = local read "Global Stop"() -> (w565:bool)
    n683 = Compound Arithmetic op=OR(w558, w563, w565) -> (w564:bool)
  }
  n684 = while {
    tunnel: w6 -> [w1456]
    tunnel: [w1457] -> _
    stop <- w1460 stop-if-true
    n685 = property on="3dAbelFcs" class="Bool (strict)"(error in=w1456) -> (error out=w1458:errorcluster, "Value"=w1459:bool)  [unwired: 1 in, 1 out]
    n686 = local read "Global Stop"() -> (w1460:bool)
    n687 = case shown="False" w1459 {
      tunnel: w1458 -> [_ w1469]
      tunnel: [_ w1475] -> w1457
      frame #0 {
      }
      frame #1 {
        n688 = local read "Z Stepsize"() -> (w1472:dbl)
        n689 = local read "Y Stepsize"() -> (w1473:dbl)
        n690 = local read "X Stepsize"() -> (w1474:dbl)
        n691 = local read "Z Steps"() -> (w1471:dbl)
        n692 = call "SetShutter.vi"("type"=T17 ?, "mode"=T18 ?, "error in (no error)"=w1469) -> ("error out"=w1461:errorcluster)  [unwired: 11 in, 1 out]
        n693 = for {
          N: w1471 -> [_]
          tunnel: w1461 -> [w1485]
          tunnel: w1472 -> [w1490]
          tunnel: w1473 -> [w1489]
          tunnel: w1474 -> [w1488]
          tunnel: [w1484] -> w1470
          tunnel: w1471 -> [w1483]
          i -> [w1487]
          n694 = local read "Z Start"() -> (w1477:dbl)
          n695 = local write "Z-Position"(w1477) -> ()
          n696 = Multiply(x=w1490, y=w1487) -> (x*y=w1481:dbl)
          n697 = Subtract(x=i32 ?, y=w1477) -> (x-y=w1478:dbl)
          n698 = local read "Y Steps"() -> (w1482:dbl)
          n699 = Add(x=w1478, y=w1481) -> (x+y=w1479:dbl)
          n700 = Number To Decimal String(number=w1487) -> (decimal integer string=w1486:string)  [unwired: 1 in]
          n701 = for {
            N: w1482 -> [_]
            tunnel: w1489 -> [w1528]
            tunnel: w1488 -> [w1527]
            tunnel: w1485 -> [w1524]
            tunnel: w1486 -> [w1526]
            tunnel: [w1498] -> w1484
            tunnel: w1477 -> [w1495]
            tunnel: w1483 -> [w1519]
            tunnel: w1482 -> [w1518]
            tunnel: w1479 -> [w1516]
            i -> [w1500]
            w1496 = string ? ("string")
            n702 = local read "X Steps"() -> (w1517:dbl)
            n703 = Number To Decimal String(number=w1500) -> (decimal integer string=w1525:string)  [unwired: 1 in]
            n704 = for {
              N: w1517 -> [_]
              tunnel: w1524 -> [w1543]
              tunnel: w1527 -> [w1548]
              tunnel: [w1544] -> w1522
              tunnel: w1526 -> [w1546]
              tunnel: w1525 -> [w1545]
              shift-right: [w1542] -> w1521
              shift-left: _ -> [w1541]
              tunnel: [w1540] -> w1520
              tunnel: [w1538] -> w1515
              tunnel: [w1539] -> w1514
              i -> [w1547]
              n705 = control-ref of="Stop Measurement"() -> (w1534:refnum<vi>)
              n706 = control-ref of="Point Measurement"() -> (w1529:refnum<vi>)
              n707 = control-ref of="Running"() -> (w1537:refnum<vi>)
              n708 = control-ref of="FCS Point Measurement"() -> (w1532:refnum<vi>)
              n709 = control-ref of="concatenated string"() -> (w1530:refnum<vi>)
              n710 = control-ref of="Workspace"() -> (w1535:refnum<vi>)
              n711 = control-ref of="X-Position"() -> (w1533:refnum<vi>)
              n712 = control-ref of="X Start"() -> (w1531:refnum<vi>)
              n713 = control-ref of="Task"() -> (w1536:refnum<vi>)
              n714 = call "LifeTimeImagePoint.vi"("Boolean in"=w1537, "String"=w1545, "reference 6"=w1533, "String 2"=w1546, "reference 7"=w1532, "error in (no error)"=w1543, "reference 4"=w1534, "reference 3"=w1535, "reference 9"=w1531, "reference in"=w1536, "Numeric in"=w1547, "Str Refnum"=w1530, "X Stepsize"=w1548, "Array in"=w1541, "Point Measurement"=w1529) -> ("Array out"=w1542:i32[][], "CCD Chip Size"=w1539:i32, "X Start"=w1540:dbl, "Numeric out"=w1538:dbl, "error out"=w1544:errorcluster)  [unwired: 8 in]
            }
            n715 = property on="Workspace" class="Path"() -> ("Value"=w1497:path)  [unwired: 2 in, 2 out]
            n716 = Increment(x=w1500) -> (x+1=w1501:i32)
            n717 = Get Date/Time In Seconds() -> (seconds since 1Jan1904=w1506:timestamp)
            n718 = Strip Path(path=w1497) -> (stripped path=w1510:path)  [unwired: 1 out]
            n719 = Format Date/Time String(time format string (%c)=string ?, seconds (now)=w1506) -> (date/time string=w1504:string)  [unwired: 1 in]
            n720 = Path To String(path=w1510) -> (string=w1511:string)
            n721 = Number To Decimal String(number=w1501) -> (decimal integer string=w1507:string)  [unwired: 1 in]
            n722 = local read "Y Start"() -> (w1491:dbl)
            n723 = local write "Y-Position"(w1491) -> ()
            n724 = Concatenate Strings(w1511, string ? ("string"), string ? ("string"), w1496, w1507, w1496, w1504, w1496, w1496) -> (w1512:string)
            n725 = Multiply(x=w1528, y=w1500) -> (x*y=w1523:dbl)
            n726 = Subtract(x=i32 ?, y=w1491) -> (x-y=w1492:dbl)
            n727 = Add(x=w1492, y=w1523) -> (x+y=w1493:dbl)
            n728 = String To Path(string=w1512) -> (path=w1503:path)
            n729 = Build Array(w1495, w1491, w1520, w1519, w1518, w1517, w1516, w1493, w1515, w1514) -> (w1513:dbl[])
            n730 = Path To String(path=w1503) -> (string=w1502:string)
            n731 = script code="results.ImagePlane=Data;\nresults.Info.Zstart=Meta(1);\nresults.Info.Ystart=Meta(2);\nresults.Info.Xstart=Meta(3);\nresults.Info.Zsteps=Meta(4);\nresults.Info.Ysteps=Meta(5);\nresults.Info.Xsteps=Meta(6);\nresults.Info.Zpos=Meta(7);\nresults.Info.Ypos=Meta(8);\nresults.Info.Xpos=Meta(9);\nresults.Info.CcdSize=Meta(13);\nsave(file,'results');\nclear results;"("??"=w1522, "Data"=w1521, "Meta"=w1513, "file"=w1502) -> ("??"=w1499:errorcluster)
            n732 = call "FreeInternalMemory.vi"("error in (no error)"=w1499) -> ("error out"=w1498:errorcluster)  [unwired: 1 in, 1 out]
          }
        }
        n733 = call "AbortAcquisition.vi"("error in (no error)"=w1470) -> ("error out"=w1467:errorcluster)  [unwired: 1 in, 1 out]
        n734 = call "SetShutter.vi"("type"=T17 ?, "mode"=T18 ?, "error in (no error)"=w1467) -> ("error out"=w1463:errorcluster)  [unwired: 11 in, 1 out]
        n735 = call <vilib>:"Clear Errors.vi"("error in (no error)"=w1463) -> ("error out"=w1462:errorcluster)  [unwired: 6 in]
        n736 = property on="3dAbelFcs" class="Bool (strict)"(error in=w1462, "Value"=bool ? ("3dAbelFcs")) -> (error out=w1475:errorcluster)  [unwired: 1 in, 1 out]
      }
    }
  }
  n737 = call "PulseTrain.vi"("error in"=w6, "duty cycle"="duty cycle", "frequency"="frequency") -> ("error out"=w5:errorcluster, "task out"=w4:refnum<k21>)  [unwired: 7 in]
  n738 = while {
    tunnel: [w1549] -> w7
    tunnel: w5 -> [w1549]
    tunnel: w4 -> [w1550]
    tunnel: [w1550] -> w3
    stop <- w1552 stop-if-true
    n739 = Wait (ms)(milliseconds to wait=u32 ?) -> ()  [unwired: 1 out]
    n740 = local read "Global Stop"() -> (w1552:bool)
  }
  n741 = call <vilib>:"DAQmx Clear Task.vi"("task in"=w3, "error in"=w7) -> ()  [unwired: 13 in, 1 out]
  n742 = global read "patternImg.vi" "New Image"() -> (w8:T5)
  n743 = call "IMAQ Dispose"("Image"=w8, "error in (no error)"=w10) -> ()  [unwired: 4 in, 1 out]
